vi "Dashboard Main.vi"() -> ()   [LabVIEW 2016]
uses:
  Vision/Camera Types.ctl
  Common Code/Drivetrain Encoder Settings.ctl
  Common Code/Drivetrain Encoder Values.ctl
  Common Code/Encoder Values.ctl
  Common Code/Drivetrain Status Cluster.ctl
  Common Code/Drivetrain Mode.ctl
  Common Code/Intake Auto States.ctl
  Common Code/Shooter Commands.ctl
  Common Code/Shot Type.ctl
  <vilib>/Rock Robotics/WPI/Camera/WPI_CameraSettings Read MJPG.ctl
  <vilib>/Rock Robotics/WPI/Camera/WPI_CameraImageSize.ctl
  Common Code/Goal Vision Packet.ctl
  Common Code/Auton Command Cluster.ctl
  Common Code/Auton File Lists.ctl
  <vilib>/Analysis/Matrix/Datatypes/RealMatrix.ctl
  Common Code/Climber Settings.ctl
  Common Code/PDP Device Currents.ctl
  Common Code/Drivetrain Settings.ctl
  Common Code/PID Gains.ctl
  Common Code/Input Modifier.ctl
  Common Code/Robot Status Cluster.ctl
  <vilib>/Rock Robotics/WPI/DriverStation/WPI_DriverStationRobotMode2.ctl
  <vilib>/Rock Robotics/WPI/DriverStation/WPI_DriverStationAllianceInfo.ctl
  <vilib>/Rock Robotics/WPI/DriverStation/WPI_DriverStationPositionInfo.ctl
  Common Code/LED Dashboard.ctl
  Common Code/Shooter Presets.ctl
  Common Code/Auto Agitator Settings.ctl
  Common Code/Shooter Motor Operational Status .ctl
  Common Code/Intake Presets.ctl
  Common Code/Shooter Status Cluster.ctl
  Common Code/Shooter Modes.ctl
  Common Code/Intake Status Cluster.ctl
  Common Code/Intake Modes.ctl
  Common Code/Intake Trip States.ctl
  Common Code/Load State.ctl
  Common Code/Unload Mode.ctl
  Common Code/Gear Vision Packet.ctl
  <vilib>/vision/Image Controls.llb/IMAQ Image.ctl
  Common Code/Dashboard Control Data.ctl
  Common Code/Vision Target Packet.ctl
  Common Code/LED Global Data.ctl
  Common Code/Robot Name.ctl
  Common Code/Dashboard Display Data.ctl
  Common Code/Climb Status Cluster.ctl
  Common Code/PDP Status Cluster.ctl
  Common Code/LED Status Cluster.ctl
  Common Code/PIXY Vision Packet.ctl
  Common Code/Utilities/Change Detect Int.vi
  <vilib>/Rock Robotics/WPI/Dashboard/WPI_DashboardLogging Global.vi
  <vilib>/Utility/inputDevices.llb/keyboardAcquire.vi
  <vilib>/vision/NI_Vision_Development_Module.lvlib
  <vilib>/Analysis/Matrix/NI_Matrix.lvlib
  <vilib>/picture/3D Picture Control/NI_3D Picture Control.lvlib
panel:
  out "Gear Vision Packet":T1
  out "Gear Front Cam":T2
  in  "Gear LED Color":T3={"Hue"={107.81818389892578, 139.81818389892578}, "Sat"={176.07142857142858, 255.0}, "Val"={40.53571428571429, 255.0}} {"Hue" scale=0.0..255.0 scale format="%#_3g"}
  in  "Gear Camera Type":T4=enum."1013"
  in  "Line Border 2":cluster{"Top":dbl, "Bottom":dbl}={"Top"=6.0, "Bottom"=1.0}
  out "DS TCP":T5
  in  "stop":bool
  in  "Rec Mode":enum32{"Stop", "Record", "Playback"}(radio)
  in  "TCP":refnum<k5>
  out "Robot IP":string
  out "Image Message":string="Timeout in Camera Communications"
  in  "Dashboard Tab":T6(tab)
  out "Pusher Activated?":bool
  out "Match Time\n(seconds)":dbl
  out "Climber Power":dbl(slide) scale=-1.0..1.0
  out "Match Time":string
  out "Current Auto Queue":string
  out "Gear?":bool
  out "back":u32(colorbox)
  out "front":u32(colorbox)
  out "Climber Tripped":bool
  out "Creep Mode?":bool
  out "Trigger Power":dbl(slide) scale=-1.0..1.0
  out "Intake Power":dbl(slide) scale=-1.0..1.0
  out "Current RPM":dbl
  out "Target RPM":dbl
  out "RPM Reached?":bool
  out "Vision Aligned?":bool
  out "Center":dbl(slide) scale=-200.0..200.0
  out "Right":dbl(slide) scale=-200.0..200.0
  out "Left":dbl(slide) scale=-200.0..200.0
  out "Target Angle Difference":dbl
  out "Distance from Target":dbl
  out "Target Found?":bool
  in  "Camera Mode 2":u16(ring) items=["Camera Off", "USB Camera SW", "USB Camera HW", "IP Camera"]
  in  "Camera Mode":u16(ring) items=["Camera Off", "USB Camera SW", "USB Camera HW", "IP Camera"]
  out "Front Camera Display":T2(plugin-control)
  out "Camera Info":cluster{"Mbps LED":bool, "Mbps":dbl, "fps":dbl} {"fps" format="%#.1g"; "Mbps" format="%#.1g"}
  out "RPM":cluster{dbl, dbl}(knob)={0.0, 114.36688146524764} scale=0.0..5000.0
  out "Traction":bool
  out "Brakes":bool
  out "Center Wheel":bool caption="Brakes"
  out "Pressure":dbl(slide) scale=0.0..120.0
  out "Wings":bool
  out "Gyro":cluster{dbl, dbl}(knob)={0.0, 101.11394868147904} scale=0.0..360.0
  out "Intake":bool
  out "Shooter":bool
  out "Shooter State":T7
  out "Shot Type":T8=enum."Dist Shot"
  out "Gear":bool
  out "Hood Down?":bool
  out "Complete Gear Load":bool
  out "Forward Tripped?":bool
  out "Backward Tripped?":bool
  out "Intake State":T9
  out "Camera Info 3":cluster{"Mbps LED":bool, "Mbps":dbl, "fps":dbl} {"fps" format="%#.1g"; "Mbps" format="%#.1g"}
  out "Robot":picture
  out "Doors Open?":bool
  out "Gear Cam":T2(plugin-control)
  in  "Drivetrain Settings":T10={"Gyro Tolerance"=1.5, "Gyro Steer PID Gains"={"proportional gain (Kc)"=0.03, "integral time (Ti, min)"=0.01, "derivative time (Td, min)"=0.0}, "Y Power Multiplier"=6.0, "Turn Power Multiplier"=5.0, "Gyro Output"=0.85, "Creep Rate"=0.4, "Distance Drive PID Gains"={"proportional gain (Kc)"=1.0, "integral time (Ti, min)"=0.01, "derivative time (Td, min)"=0.0}, "Distance Tolerance"=1.4999999999999998, "Distance Output"=0.85, "Strafe Threshold"=0.4, "Strafe Correct"=FALSE, "Strafe Tolerance"=0.0, "Translate Drive PID Gains"={"proportional gain (Kc)"=1.0, "integral time (Ti, min)"=0.01, "derivative time (Td, min)"=0.0}, "Strafe Output"=0.0, "SC Right"=0.85, "SC Left"=0.85, "Use Gyro"=FALSE, "Constant Power"=FALSE, "Strafe Power"=0.0, "Input Modifier"=enum."None", "SCR Delay"=0.85, "SCL Delay"=0.85} {"Translate Drive PID Gains"."derivative time (Td, min)" format="%.3f"; "Translate Drive PID Gains"."integral time (Ti, min)" format="%.3f"; "Translate Drive PID Gains"."proportional gain (Kc)" format="%.3f"; "Distance Drive PID Gains"."derivative time (Td, min)" format="%.3f"; "Distance Drive PID Gains"."integral time (Ti, min)" format="%.3f"; "Distance Drive PID Gains"."proportional gain (Kc)" format="%.3f"; "Turn Power Multiplier" scale=0.0..6.0; "Y Power Multiplier" scale=0.0..6.0; "Gyro Steer PID Gains"."derivative time (Td, min)" format="%.3f"; "Gyro Steer PID Gains"."integral time (Ti, min)" format="%.3f"; "Gyro Steer PID Gains"."proportional gain (Kc)" format="%.3f"}
  in  "Zero Gyro":bool
  in  "Drivetrain Encoder Settings":T13
  out "Drivetrain Encoder Values":T14
  out "Drivetrain Status Cluster":T16={"Y (Throttle)"=0.0, "X (Steer)"=0.0, "Z (Strafe)"=0.0, "Heading Target"=0.0, "Center Piston Down?"=FALSE, "Traction?"=FALSE, "Gyro Steer Finished?"=FALSE, "Distance Drive Finished?"=FALSE, "Gyro"=0.0, "Distance Target"=0.0, "Y Max Output"=0.0, "Y Min Output"=0.0, "X Max Output"=0.0, "X Min Output"=0.0, "Z Max Output"=0.0, "Z Min Output"=0.0, "Translation Target"=0.0, "Translation Drive Finished?"=FALSE, "PID Auto Drive Finished?"=FALSE, "Brake?"=FALSE, "Vision Aligned?"=FALSE, "Creep Mode Engaged?"=FALSE, "Drivetrain Mode"=enum."Gyro Steer", "Gear Vision Aligned?"=FALSE} {"Gyro" scale=180.0..-180.0}
  out "Intake Status Cluster":T18={"Roller Power"=0.0, "Intake Mode"=enum."Manual", "Intake Auto State"=enum."Idle", "Backward Tripped?"=FALSE, "Forward Tripped?"=FALSE, "Intake Current Trip State"=enum."Normal", "Gear Flap Open"=FALSE, "Doors Open"=FALSE, "Traction for Gear?"=FALSE, "Current"=0.0, "Intake Down?"=FALSE, "Gear Loaded"=FALSE, "Pusher Activated"=FALSE, "Gear Load State"=enum."Idle", "Unload Mode"=enum."None", "Unloading Gear?"=FALSE}
  out "Shooter Status Cluster":T23={"Current RPM"=0.0, "Trigger Power"=0.0, "Shooter Mode"=enum."Auto", "Shot Type"=enum."Dist Shot", "Shooter State"=enum."Idle ", "Target RPM"=0.0, "Hood Down?"=FALSE, "RPM Reached?"=FALSE, "User Inputed RPM"=0.0} {"Current RPM" scale=0.0..5000.0}
  in  "Intake Presets":T25
  out "Motor Operational Status":T26
  in  "Auto Agitator":T27
  in  "Shooter Presets":T28
  out "Distance Shots":T29
  in  "Particles":dbl=5.0
  in  "Camera Settings":T30={"fps"=30, "compression"=30, "Image Size"=enum."320x240", "Config Shown"=FALSE}
  out "Original Image":T2(plugin-control)
  in  "Camera Type":T4=enum."1013"
  in  "Line Border":cluster{"Top":dbl, "Bottom":dbl}={"Top"=6.0, "Bottom"=1.0}
  in  "Use Calibration":bool=TRUE
  in  "Score Cutoff %":dbl=70.0
  out "Qualified Particles":i32
  in  "LED Color":T3={"Hue"={107.81818389892578, 139.81818389892578}, "Sat"={176.07142857142858, 255.0}, "Val"={40.53571428571429, 255.0}} {"Hue" scale=0.0..255.0 scale format="%#_3g"}
  out "Results":T32 {"Score" format="%#_3g"; "Pixels"."Rectangle"."Numeric 5" format="%#_3g"; "Pixels"."Rectangle"."Numeric 3" format="%#_3g"; "Pixels"."Rectangle"."Numeric 2" format="%#_3g"; "Pixels"."Rectangle"."Numeric" format="%#_3g"; "Normalized"."Rectangle"."Numeric 5" format="%#_2g"; "Normalized"."Rectangle"."Numeric 3" format="%#_2g"; "Normalized"."Rectangle"."Numeric 2" format="%#_2g"; "Normalized"."Rectangle"."Numeric" format="%#_2g"; "Normalized"."Center"."?" format="%#_3g"; "Normalized"."Center"."?" format="%#_3g"; "Distance (ft)" format="%#_3g"}
  out "Masked Image":T2(plugin-control)
  out "Goal Vision Packet":T33
  in  "Vision Timeout":dbl=70.0
  out "Gear Results":T32 {"Score" format="%#_3g"; "Pixels"."Rectangle"."Numeric 5" format="%#_3g"; "Pixels"."Rectangle"."Numeric 3" format="%#_3g"; "Pixels"."Rectangle"."Numeric 2" format="%#_3g"; "Pixels"."Rectangle"."Numeric" format="%#_3g"; "Normalized"."Rectangle"."Numeric 5" format="%#_2g"; "Normalized"."Rectangle"."Numeric 3" format="%#_2g"; "Normalized"."Rectangle"."Numeric 2" format="%#_2g"; "Normalized"."Rectangle"."Numeric" format="%#_2g"; "Normalized"."Center"."?" format="%#_3g"; "Normalized"."Center"."?" format="%#_3g"; "Distance (ft)" format="%#_3g"}
  out "Gear Qualified Particles":i32
  in  "Gear Score Cutoff %":dbl=70.0
  in  "Gear Use Calibration":bool=TRUE
  out "Gear Original Image":T2(plugin-control)
  out "Gear Masked Image":T2(plugin-control)
  in  "Particles 2":dbl=5.0
  in  "Gear Camera Settings":T30={"fps"=30, "compression"=30, "Image Size"=enum."320x240", "Config Shown"=FALSE}
  in  "Gear Vision Packet 2":T1
  out "Auton File Lists":T34
  out "Auton Command Cluster":T35
  in  "Auton Presets":cluster{"Start Position":dbl}
  in  "LEDs":T36
  out "Robot Status Cluster":T37
  in  "Robot Photos Folder":path=path "C:/Users/Team624/Desktop/SteamyRobot/Dashboard/Dashboard Nautilus"
  out "Climber Current Tripped":bool
  in  "Climber Settings":T41
  in  "Pressure M":dbl
  in  "Pressure B":dbl
  out "Pressure":dbl
  out "Pressure Voltage":dbl
  out "Total Current":dbl
  out "PDP Currents":T42
  out "Status Info":T43
  out "Control Info":T44
  out "Robot Metrics":T45
  out "Shooter RPM History":dbl(graph)
  in  "Open in Excel":bool
  in  "Save":bool
  in  "Load":bool
  out "DumbDashMessage":string
  # "CRyptonite Robotics DumbDashboard 2k17"
  # "Drivetrain"
  # "Collection"
  # "Drivetrain Speeds"
  # "Driver\nA0 - none\nA1 - Throttle\nA2 - Strafe Left\nA3 - Strafe Right\nA4 - Turn\nA5 - none\n\nB0 - Vision Align (Hold)\nB1 - none\nB2 - none\nB3 - Brakes (Hold)\nB4 - Creep Mode (Hold)\nB5 - Traction (Toggle)\nB6 - none\nB7 - none\nB8 - none\nB9 - none\n\nU - none\nD - none\nL - Gyro Steer Left (Hold)\nR - Gyro Steer Right (Hold)"
  # "Manipulator\nA0 - none\nA1 - Manual Shooter Power\nA2 - Outtake\nA3 - Intake\nA4 - none\nA5 - Manual Trigger Power\n\nB0 - Shoot (Hold)\nB1 - Change Intake Mode (Toggle)\nB2 - Warmup Shooter (Hold)\nB3 - Change Shooter Mode (Toggle)\nB4 - Engage Traction for Gear (Hold)\nB5 - Manual Hood (Toggle)\nB6 - Agitator (Hold)\nB7 - Climb\nB8 - Open Gear Flap (Hold)\nB9 - Open Wings (Hold)\n\nU - none\nD - none\nL - Distance Shot Type (1 Way Toggle)\nR - Key Shot Type (1 Way Toggle"
  # "A2"
  # "A3"
  # "B4"
  # "B5"
  # "B6"
  # "B7"
  # "B3"
  # "U"
  # "B2"
  # "B1"
  # "L"
  # "R"
  # "A5"
  # "A1"
  # "B0"
  # "D"
  # "A0"
  # "A4"
  # "B8"
  # "B9"
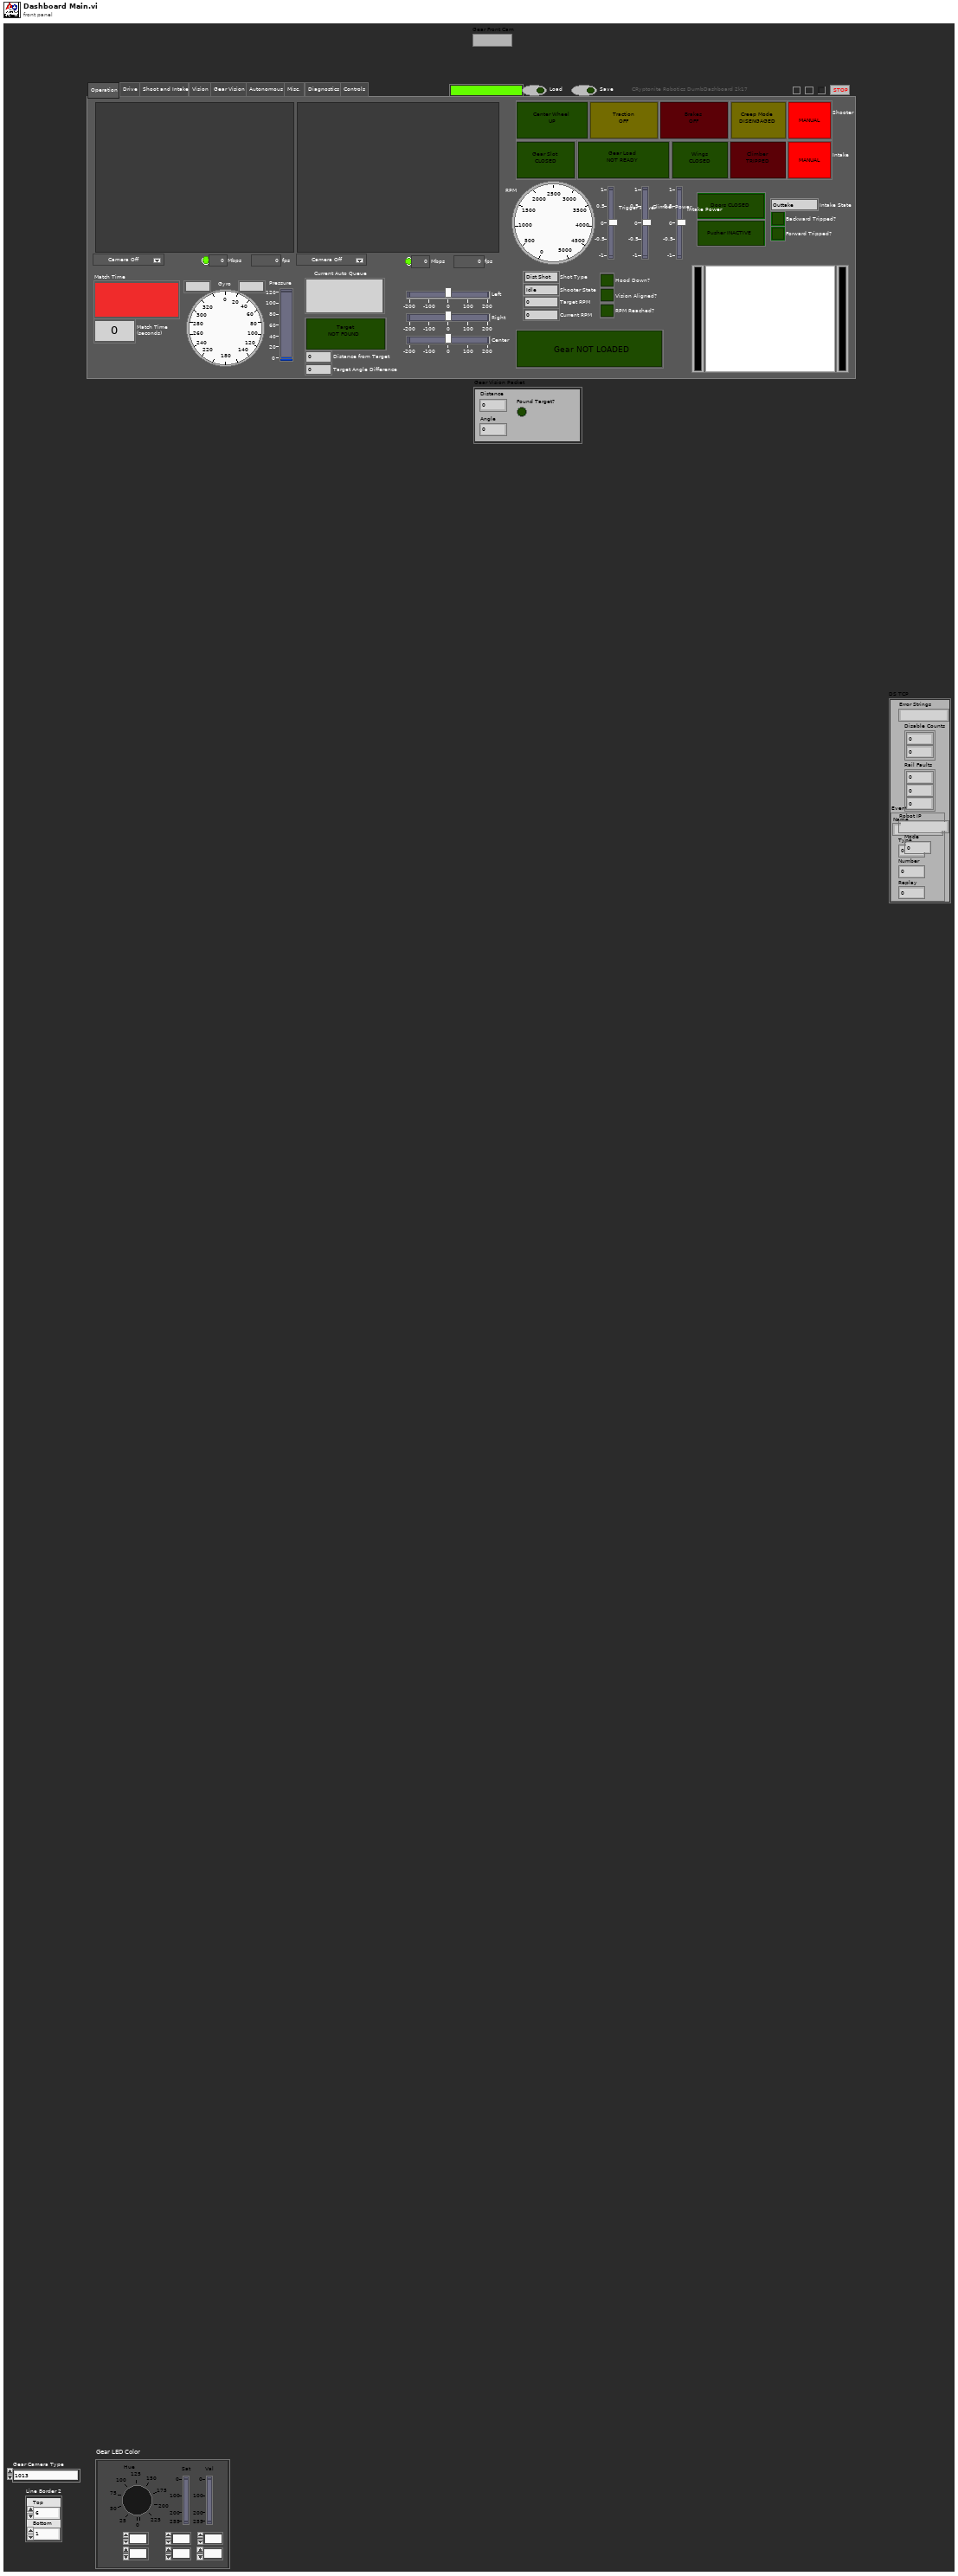
[diagram p1: front panel]
types:
  T1 = typedef "Gear Vision Packet.ctl" = cluster{"Distance":dbl, "Angle":dbl, "Found Target?":bool}
  T2 = typedef "IMAQ Image.ctl" = refnum<image>
  T3 = cluster{"Hue":cluster{dbl, dbl}, "Sat":cluster{dbl, dbl}, "Val":cluster{dbl, dbl}}
  T4 = typedef "Camera Types.ctl" = enum16{"206", "1011", "1013", "MS HD3000 square", "MS HD3000 640x480"}
  T5 = cluster{"Error Strings":string, "Disable Counts":cluster{u16, u16}, "Rail Faults":cluster{u16, u16, u16}, "Robot IP":string, "Mode":u8, "Event Info":cluster{"Name":string, "Type":u8, "Number":u16, "Replay":u8}}
  T6 = enum32{"Operation", "Drive", "Shoot and Intake", "Vision", "Gear Vision", "Autonomous", "Misc.", "Diagnostics", "Controls"}
  T7 = typedef "Shooter Commands.ctl" = enum16{"Idle ", "Warmup ", "Shoot"}
  T8 = typedef "Shot Type.ctl" = enum16{"Vision Shot", "Dist Shot", "Key Shot"}
  T9 = typedef "Intake Auto States.ctl" = enum16{"Outtake", "Idle", "Intake", "Intake Pull Up"}
  T10 = typedef "Drivetrain Settings.ctl" = cluster{"Gyro Tolerance":dbl, "Gyro Steer PID Gains":T11, "Y Power Multiplier":dbl, "Turn Power Multiplier":dbl, "Gyro Output":dbl, "Creep Rate":dbl, "Distance Drive PID Gains":T11, "Distance Tolerance":dbl, "Distance Output":dbl, "Strafe Threshold":dbl, "Strafe Correct":bool, "Strafe Tolerance":dbl, "Translate Drive PID Gains":T11, "Strafe Output":dbl, "SC Right":dbl, "SC Left":dbl, "Use Gyro":bool, "Constant Power":bool, "Strafe Power":dbl, "Input Modifier":T12, "SCR Delay":dbl, "SCL Delay":dbl}
  T11 = typedef "PID Gains.ctl" = cluster{"proportional gain (Kc)":dbl, "integral time (Ti, min)":dbl, "derivative time (Td, min)":dbl}
  T12 = typedef "Input Modifier.ctl" = enum16{"None", "Square", "Cube"}
  T13 = typedef "Drivetrain Encoder Settings.ctl" = cluster{"Left Tick Constant":dbl, "Right Tick Contant":dbl, "Reset Encoders":bool, "Center Tick Constant":dbl}
  T14 = typedef "Drivetrain Encoder Values.ctl" = cluster{"Left Encoder":T15, "Center Encoder":T15, "Right Encoder":T15}
  T15 = typedef "Encoder Values.ctl" = cluster{"Distance":dbl, "Speed":dbl, "Tick":dbl}
  T16 = typedef "Drivetrain Status Cluster.ctl" = cluster{"Y (Throttle)":dbl, "X (Steer)":dbl, "Z (Strafe)":dbl, "Heading Target":dbl, "Center Piston Down?":bool, "Traction?":bool, "Gyro Steer Finished?":bool, "Distance Drive Finished?":bool, "Gyro":dbl, "Distance Target":dbl, "Y Max Output":dbl, "Y Min Output":dbl, "X Max Output":dbl, "X Min Output":dbl, "Z Max Output":dbl, "Z Min Output":dbl, "Translation Target":dbl, "Translation Drive Finished?":bool, "PID Auto Drive Finished?":bool, "Brake?":bool, "Vision Aligned?":bool, "Creep Mode Engaged?":bool, "Drivetrain Mode":T17, "Gear Vision Aligned?":bool}
  T17 = typedef "Drivetrain Mode.ctl" = enum16{"Gear Vision Align", "Manual", "Gyro Steer", "Distance Drive", "Translate Drive", "Goal Vision Align", "PID Drive"}
  T18 = typedef "Intake Status Cluster.ctl" = cluster{"Roller Power":dbl, "Intake Mode":T19, "Intake Auto State":T9, "Backward Tripped?":bool, "Forward Tripped?":bool, "Intake Current Trip State":T20, "Gear Flap Open":bool, "Doors Open":bool, "Traction for Gear?":bool, "Current":dbl, "Intake Down?":bool, "Gear Loaded":bool, "Pusher Activated":bool, "Gear Load State":T21, "Unload Mode":T22, "Unloading Gear?":bool}
  T19 = typedef "Intake Modes.ctl" = enum16{"Manual", "Auto"}
  T20 = typedef "Intake Trip States.ctl" = enum16{"Normal", "Backward Tripped", "Forward Tripped"}
  T21 = typedef "Load State.ctl" = enum16{"Idle", "Open Flap", "Ready Close", "Ready Far"}
  T22 = typedef "Unload Mode.ctl" = enum16{"None", "Close", "Far"}
  T23 = typedef "Shooter Status Cluster.ctl" = cluster{"Current RPM":dbl, "Trigger Power":dbl, "Shooter Mode":T24, "Shot Type":T8, "Shooter State":T7, "Target RPM":dbl, "Hood Down?":bool, "RPM Reached?":bool, "User Inputed RPM":dbl}
  T24 = typedef "Shooter Modes.ctl" = enum16{"Auto", "Manual"}
  T25 = typedef "Intake Presets.ctl" = cluster{"Intake Speed ":dbl, "Outake Speed":dbl, "Current Trip Delay":dbl, "Max Current":dbl, "Gear Outtake Motor Delay":dbl, "Gear Intake Motor Delay":dbl, "Gear Intake Pull Up Speed":dbl, "Pusher Delay":dbl, "Release Delay":dbl, "Close Release Delay":dbl}
  T26 = typedef "Shooter Motor Operational Status .ctl" = cluster{"Sensor Velocity ":dbl, "Encoder Position":dbl, "Encoder Velocity ":dbl, "Encoder Index Count":dbl, "Analog In":dbl, "Analog In Velocity":dbl, "Battery Voltage":dbl, "Current":dbl, "Sensor Position":dbl, "Vel Div 4":bool, "Encoder A Pin State":bool, "Encoder B Pin State":bool, "Encoder Index Pin State":bool, "Pulse Width Velocity ":dbl}
  T27 = typedef "Auto Agitator Settings.ctl" = cluster{"Enable Auto Agitation":bool, "Continuous Stir":bool, "Continuous Intake":bool, "Alternate In/Outtake":bool, "Wing Delay":dbl, "Stir Delay":dbl, "Intake Delay":dbl, "Wing On Time":dbl, "Wing Off Time":dbl, "Stir On Time":dbl, "Stir Off Time":dbl, "Intake On Time":dbl, "Intake Off Time":dbl, "Stir Power":dbl, "Intake Power":dbl, "Outtake Power":dbl, "Intake Run Time":dbl, "Outtake Run Time":dbl, "Wing$":bool, "Intake":bool, "Stirrer":bool}
  T28 = typedef "Shooter Presets.ctl" = cluster{"Key Shot":cluster{"RPM ":dbl, "Hood?":bool}, "Distance Shot":cluster{"RPM":dbl, "Hood?":bool}, "RPM Tolerance":dbl, "Unstuck Delay Time ":dbl, "Initial RPM Increase":dbl, "Warmup Delay":dbl, "Faster Time":dbl, "Shooter PID Gains":cluster{"P":dbl, "I":dbl, "D":dbl, "FF":dbl, "Ramp Rate":dbl, "I Zone":dbl}, "Unstuck Trigger Power":dbl, "Trigger Power":dbl, "Unstuck RPM":dbl, "Agitator Active Power":dbl, "Agitator Idle Power":dbl, "RPM Tuning Range":dbl, "RPM M Tuning Range":dbl}
  T29 = typedef "NI_Matrix.lvlib/RealMatrix.ctl" = dbl[][]
  T30 = typedef "WPI_CameraSettings Read MJPG.ctl" = cluster{"fps":i32, "compression":i32, "Image Size":T31, "Config Shown":bool}
  T31 = typedef "WPI_CameraImageSize.ctl" = enum16{"640x480", "320x240", "160x120", "Custom"}
  T32 = cluster{"Distance (ft)":dbl, "Score":dbl, "Normalized":cluster{"Center":cluster{dbl, dbl}, "Rectangle":cluster{"Numeric":dbl, "Numeric 2":dbl, "Numeric 3":dbl, "Numeric 5":dbl}}, "Pixels":cluster{"Center":cluster{dbl, dbl}, "Rectangle":cluster{"Numeric":dbl, "Numeric 2":dbl, "Numeric 3":dbl, "Numeric 5":dbl}}}
  T33 = typedef "Goal Vision Packet.ctl" = cluster{"Distance":dbl, "Angle":dbl, "Found Target?":bool}
  T34 = typedef "Auton File Lists.ctl" = cluster{"Current Queue":string, "General Scripts":string, "Movements":string}
  T35 = typedef "Auton Command Cluster.ctl" = cluster{"commandID":dbl, "maxTime":dbl, "distanceTarget":dbl, "headingTarget":dbl, "translationTarget":dbl, "ySpeed":dbl, "xSpeed":dbl, "zSpeed":dbl, "async":dbl, "shotType":dbl, "shootCommand":dbl, "rollerPower":dbl, "fillHopper?":dbl, "zeroGyro":dbl, "openGear":dbl, "traction?":dbl}
  T36 = typedef "LED Dashboard.ctl" = cluster{"Back":cluster{"Default":string, "Gear Ready Close":string, "Break On":string, "Gear Loaded":string, "Traction":string, "Climb":string, "Gear Ready Far":string, "Unload Gear":string, "Prime Unload":string}, "LEDOnTime":dbl, "LEDOffTime":dbl, "Front":cluster{"Default":string, "Traction":string, "Gear Ready Close":string, "Break On":string, "Gear Loaded":string, "Climb":string, "Gear Ready Far":string, "Unload Gear":string, "Prime Unload":string}}
  T37 = typedef "Robot Status Cluster.ctl" = cluster{"RobotMode":T38, "Alliance":T39, "Position":T40, "Match Time":dbl, "FMS?":bool}
  T38 = typedef "WPI_DriverStationRobotMode2.ctl" = enum16{"Autonomous Disabled", "Autonomous Enabled", "Teleop Disabled", "Teleop Enabled", "Disconnected", "Finish", "Test Disabled", "Test Enabled", "Emergency Stopped"}
  T39 = typedef "WPI_DriverStationAllianceInfo.ctl" = enum16{"Red", "Blue", "Invalid"}
  T40 = typedef "WPI_DriverStationPositionInfo.ctl" = enum16{"1", "2", "3"}
  T41 = typedef "Climber Settings.ctl" = cluster{"Climber Power":dbl, "Max Current":dbl, "Avoid Current Trip?":bool}
  T42 = typedef "PDP Device Currents.ctl" = cluster{"Drivetrain Left CIM 1":dbl, "Drivetrain Left CIM 2":dbl, "Drivetrain Left Mini CIM":dbl, "Drivetrain Right CIM 1":dbl, "Drivetrain Right CIM 2":dbl, "Drivetrain Right Mini CIM":dbl, "Drivetrain Center CIM 1":dbl, "Drivetrain Center CIM 2":dbl, "Shooter Motor 1":dbl, "Shooter Motor 2":dbl, "Climber Motor 1":dbl, "Climber Motor 2":dbl, "Intake Motor":dbl, "Trigger Motor":dbl, "Fans/Compressor":dbl}
  T43 = cluster{"Status bits":cluster{"Test Mode":bool, "Autonomous":bool, "Enabled":bool, "Code Start":bool, "Brownout":bool, "Reserved 2":bool, "Reserved 3":bool, "E-Stop":bool}, "Code Trace":cluster{"Disabled":bool, "TeleOp":bool, "Auto":bool, "Test":bool}, "Controller Type":enum16{"unknown", "cRIO", "roboRio"}, "Code?":enum16{"unknown", "noCode", "code"}, "Battery V":dbl}
  T44 = cluster{"Control Bits":cluster{"TestMode":bool, "Autonomous":bool, "Enabled":bool, "FMS Present":bool, bool, bool, bool, "E-Stop":bool}, "Team Station ":u8, "Countdown":sgl, "Joystick Values":cluster{"Axes":dbl[], "Buttons":bool[], "POVs":i16[]}[]}
  T45 = cluster{"Storage":cluster{"Disk Free":u64, "RAM Block":u32, "RAM free":u32}, "CPU Utilization":cluster{"CPU % ISR":sgl, "CPU % Time Crit":sgl, "CPU % Timed Str":sgl, "CPU % High":sgl, "CPU % Above":sgl, "CPU % Normal":sgl, "CPU % Low":sgl}, "CAN":cluster{"% Bus Utilization":sgl, "Bus Off Cnt":u32, "TX_FIFO Full Cnt":u32, "Receive Error Cnt":u8, "Transmit Error Cnt":u8}, "HID":cluster{"HID Outputs":u32, "Rumble Low":u16, "Rumble High":u16}[]}
  T46 = typedef "Image Type" = u32
  T47 = typedef "Particle Parameters" = i32
  T48 = cluster{"IDs":cluster{"RPC field ID":u16, "Unique ID":u16}, "String":string}
  T49 = enum32{"Drive", "Basic", "Custom", "Test", "Checklist", "Variables"}
  T50 = typedef "LED Global Data.ctl" = cluster{"Back":cluster{"Default":string, "Traction":string, "Gear Ready Close":string, "Break On":string, "Gear Loaded":string, "Climb":string, "Gear Ready Far":string, "Unload Gear":string, "Prime Unload":string}, "Front":cluster{"Default":string, "Traction":string, "Gear Ready Close":string, "Break On":string, "Gear Loaded":string, "Climb":string, "Gear Ready Far":string, "Unload Gear":string, "Prime Unload":string}, "LEDOnTime":dbl, "LEDOffTime":dbl}
  T51 = typedef "Dashboard Control Data.ctl" = cluster{"Drivetrain Settings":T10, "Intake Presets ":T25, "Shooter Presets":T28, "Vision Target Packet":T52, "Auton Presets":cluster{"Start Position":dbl}, "Drivetrain Encoder Values":T14, "Drivetrain Encoder Settings":cluster{"Left Tick Constant":dbl, "Right Tick Contant":dbl, "Reset Encoders":bool, "Center Tick Constant":dbl}, "Zero Gyro":bool, "Vision Timeout":dbl, "Pressure M":dbl, "Pressure B":dbl, "Auto Agitator":T27, "Climber Settings":T41, "LEDs":T50}
  T52 = typedef "Vision Target Packet.ctl" = cluster{"Robot Center":dbl, "Center X":dbl, "Center Y":dbl, "Angle":dbl, "Distance":dbl, "Found Target?":bool}
  T53 = cluster{cluster{dbl, dbl}, cluster{dbl, dbl}, cluster{dbl, dbl}}
  T54 = cluster{"Left":dbl, "Top":dbl, "Right":dbl, "Bottom":dbl}
  T55 = cluster{"Numeric":dbl, "Numeric 2":dbl, "Numeric 3":dbl, "Numeric 5":dbl}
  T56 = enum16{"0", "1", "2", "3", "4", "5", "6", "7", "8", "9", "A", "B", "C", "D", "E", "F", "G", "H", "I", "J", "K", "L", "M", "N", "O", "P", "Q", "R", "S", "T", "U", "V", "W", "X", "Y", "Z", "F1", "F2", "F3", "F4", "F5", "F6", "F7", "F8", "F9", "F10", "F11", "F12", "F13", "F14", "F15", "ADD", "BACK", "BACKSLASH", "CAPITAL", "COMMA", "DECIMAL", "DELETE", "DIVIDE", "DOWN", "END", "EQUALS", "ESCAPE", "GRAVE (`)", "HOME", "INSERT", "LBRACKET", "LCONTROL", "LEFT", "L ALT", "LSHIFT", "LWIN", "MINUS", "MULTIPLY", "NEXT", "NUMLOCK", "NUMPAD_0", "NUMPAD_1", "NUMPAD_2", "NUMPAD_3", "NUMPAD_4", "NUMPAD_5", "NUMPAD_6", "NUMPAD_7", "NUMPAD_8", "NUMPAD_9", "PAUSE", "PERIOD", "PRIOR (PG UP)", "RBRACKET", "RCONTROL", "RETURN", "RIGHT", "R ALT", "RSHIFT", "RWIN", "SCROLL", "SEMICOLON", "SLASH", "SPACE", "SUBTRACT", "TAB", "UP", "ENTER (num pad)", "' (quote)"}
  T57 = enum16{"0", "1", "2", "3", "4", "5", "6", "7", "8", "9", "A", "B", "C", "D", "E", "F", "G", "H", "I", "J", "K", "L", "M", "N", "O", "P", "Q", "R", "S", "T", "U", "V", "W", "X", "Y", "Z", "F1", "F2", "F3", "F4", "F5", "F6", "F7", "F8", "F9", "F10", "F11", "F12", "F13", "F14", "F15", "ADD", "BACK", "BACKSLASH", "CAPITAL", "COMMA", "DECIMAL", "DELETE", "DIVIDE", "DOWN", "END", "EQUALS", "ESCAPE", "GRAVE (`)", "HOME", "INSERT", "LBRACKET", "LCONTROL", "LEFT", "L ALT", "LSHIFT", "LWIN", "MINUS", "MULTIPLY", "NEXT", "NUMLOCK", "NUMPAD_0", "NUMPAD_1", "NUMPAD_2", "NUMPAD_3", "NUMPAD_4", "NUMPAD_5", "NUMPAD_6", "NUMPAD_7", "NUMPAD_8", "NUMPAD_9", "PAUSE", "PERIOD", "PRIOR (PG UP)", "RBRACKET", "RCONTROL", "RETURN", "RIGHT", "R ALT", "RSHIFT", "RWIN", "SCROLL", "SEMICOLON", "SLASH", "SPACE", "SUBTRACT", "TAB", "UP", "ENTER (num pad)", "' (quote)"}[]
  T58 = typedef "Dashboard Display Data.ctl" = cluster{"Climb Status Cluster":T59, "Drivetrain Status Cluster":T16, "Intake Status Cluster":T18, "Shooter Status Cluster":T23, "Drivetrain Encoder Values":T14, "Auton Command Cluster":T35, "Auton File Lists":T34, "Pressure":dbl, "Pressure Voltage":dbl, "Motor Operational Status":T26, "Vision Presets":T29, "Climber Current Tripped?":bool, "Gear?":bool, "PDP Status Cluster":T60, "Robot Status Cluster":T37, "LED Status Cluster":T61, "PIXY Vision Packet":T62}
  T59 = typedef "Climb Status Cluster.ctl" = cluster{"Climb Speed":dbl}
  T60 = typedef "PDP Status Cluster.ctl" = cluster{"Drivetrain Left CIM 1":dbl, "Drivetrain Left CIM 2":dbl, "Drivetrain Left Mini CIM":dbl, "Drivetrain Right CIM 1":dbl, "Drivetrain Right CIM 2":dbl, "Drivetrain Right Mini CIM":dbl, "Drivetrain Center CIM 1":dbl, "Drivetrain Center CIM 2":dbl, "Shooter Motor 1":dbl, "Shooter Motor 2":dbl, "Climber Motor 1":dbl, "Climber Motor 2":dbl, "Intake Motor":dbl, "Trigger Motor":dbl, "Fans/Compressor":dbl}
  T61 = typedef "LED Status Cluster.ctl" = cluster{"Front Red":bool, "Front Green":bool, "Front Blue":bool, "Back Red":bool, "Back Green":bool, "Back Blue":bool}
  T62 = typedef "PIXY Vision Packet.ctl" = cluster{"Objects":cluster{"Signature":u16, "X Position":u16, "Y Position":u16, "Width":u16, "Height":u16}[]}
  T63 = enum8{"Tele-Op Disabled", "Tele-Op Enabled", "Auto Disabled", "Auto Enabled", "Test Disabled", "Test Enabled", "Disconnected", "No Code", "E-Stop"}
  T64 = typedef "LVDateTimeRec.ctl" = cluster{"fractional second":dbl, "second":i32, "minute":i32, "hour":i32, "day of month":i32, "month":i32, "year":i32, "day of week":i32, "day of year":i32, "DST":i32}
  T65 = typedef "imagedata.ctl" = cluster{"image type":i32, "image depth":i32, "image":u8[], "mask":u8[], "colors":u32[], "Rectangle":cluster{"left":i16, "top":i16, "right":i16, "bottom":i16}}
  T66 = cluster{"Image Size":bool, "Image Type":bool, "Pixel Value":bool, "ROI Information":bool, "Zoom Factor":bool}
  T67 = typedef "DumbDash Control.ctl" = cluster{"Name":string, "Ref":refnum<vi>, "Type":T68}
  T68 = typedef "DumbDash Control Type.ctl" = enum16{"Invalid", "Number", "Boolean", "String"}
  T69 = typedef "Robot Name.ctl" = u16
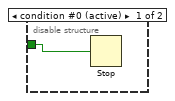
[diagram p5: hidden frame]
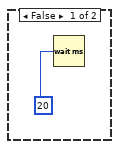
[diagram p6: hidden frame]
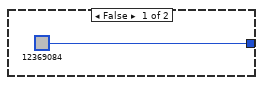
[diagram p9: hidden frame]
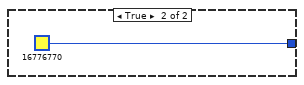
[diagram p10: hidden frame]
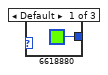
[diagram p13: hidden frame]
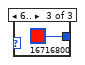
[diagram p14: hidden frame]
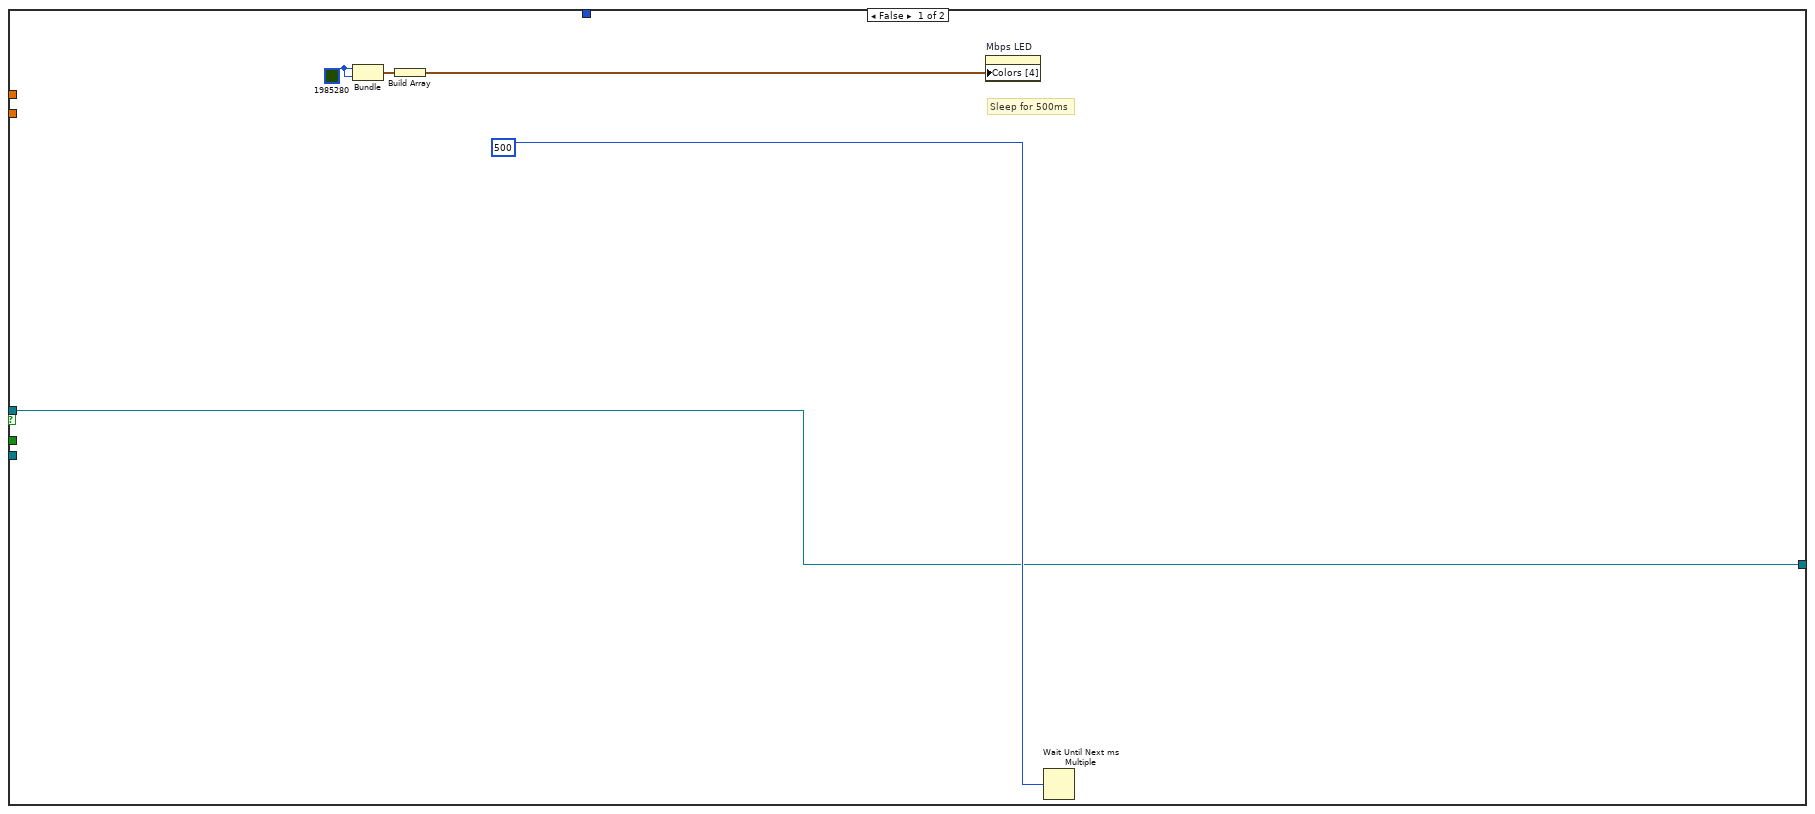
[diagram p15: hidden frame]
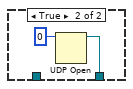
[diagram p16: hidden frame]
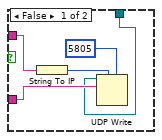
[diagram p17: hidden frame]
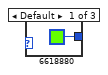
[diagram p19: hidden frame]
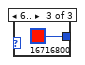
[diagram p20: hidden frame]
diagram:
  w3 = T46 4 items=["Grayscale (U8)", "Grayscale (I16)", "Grayscale (SGL)", "Complex (CSG)", "RGB (U32)", "HSL (U32)", "RGB (U64)"] ("Image Type")
  w6 = T46 4 items=["Grayscale (U8)", "Grayscale (I16)", "Grayscale (SGL)", "Complex (CSG)", "RGB (U32)", "HSL (U32)", "RGB (U64)"] ("Image Type")
  w9 = T46 0 items=["Grayscale (U8)", "Grayscale (I16)", "Grayscale (SGL)", "Complex (CSG)", "RGB (U32)", "HSL (U32)", "RGB (U64)"] ("Image Type")
  w14 = enum32{"Stop", "Record", "Playback"}."Stop" ("Rec Mode")
  w21 = T47[] [48, 35, 4, 5, 6, 7, 0, 1] items=["Center of Mass X", "Center of Mass Y", "First Pixel X", "First Pixel Y", "Bounding Rect Left", "Bounding Rect Top", "Bounding Rect Right", "Bounding Rect Bottom", "Max Feret Diameter Start X", "Max Feret Diameter Start Y", "Max Feret Diameter End X", "Max Feret Diameter End Y", "Max Horiz. Segment Length Left", "Max Horiz. Segment Length Right", "Max Horiz. Segment Length Row", "-", "Bounding Rect Width", "Bounding Rect Height", "Bounding Rect Diagonal", "Perimeter", "Convex Hull Perimeter", "Holes' Perimeter", "Max Feret Diameter", "Equivalent Ellipse Major Axis", "Equivalent Ellipse Minor Axis", "Equivalent Ellipse Minor Axis (Feret)", "Equivalent Rect Long Side", "Equivalent Rect Short Side", "Equivalent Rect Diagonal", "Equivalent Rect Short Side (Feret)", "Average Horiz. Segment Length", "Average Vert. Segment Length", "Hydraulic Radius", "Waddel Disk Diameter", "-", "Area", "Holes' Area", "Particle & Holes' Area", "Convex Hull Area", "Image Area", "-", "Number of Holes", "Number of Horiz. Segments", "Number of Vert. Segments", "-", "Orientation", "Max Feret Diameter Orientation", "-", "% Area/Image Area", "% Area/(Particle & Holes' Area)", "Ratio of Equivalent Ellipse Axes", "Ratio of Equivalent Rect Sides", "-", "Elongation Factor", "Compactness Factor", "Heywood Circularity Factor", "Type Factor", "-", "Sum X", "Sum Y", "Sum XX", "Sum XY", "Sum YY", "Sum XXX", "Sum XXY", "Sum XYY", "Sum YYY", "-", "Moment of Inertia XX", "Moment of Inertia XY", "Moment of Inertia YY", "Moment of Inertia XXX", "Moment of Inertia XXY", "Moment of Inertia XYY", "Moment of Inertia YYY", "Norm. Moment of Inertia XX", "Norm. Moment of Inertia XY", "Norm. Moment of Inertia YY", "Norm. Moment of Inertia XXX", "Norm. Moment of Inertia XXY", "Norm. Moment of Inertia XYY", "Norm. Moment of Inertia YYY", "Hu Moment 1", "Hu Moment 2", "Hu Moment 3", "Hu Moment 4", "Hu Moment 5", "Hu Moment 6", "Hu Moment 7"] ("Pixel Measurements")
  w25 = T48 {"IDs"={"RPC field ID"=0, "Unique ID"=0}, "String"=""}  # RPC Response
  w31 = 491  # min tab size
  w30 = 1.333  # min tab size
  (unwired) "This VI has seven parallel loops for different tasks and a bit of initialization code that runs just once.\n\nTypical dashboard extensions only need to edit the panel. Adding new indicators or controls simply involves placing them on the panel in the Operations tab and naming them the same as the SmartDashboard variable on the robot\n\nIf the display needs to process the data before display, loop one is an example of doing that for the joysticks and motors.\n\nIf you want customize the video display or perform processing on it, loop two is where that takes place.\n\nOther loops should not need to be modified. They are pretty standard, and document the task they perform."  # Documentation
  w46 = T46 4 items=["Grayscale (U8)", "Grayscale (I16)", "Grayscale (SGL)", "Complex (CSG)", "RGB (U32)", "HSL (U32)", "RGB (U64)"] ("Image Type")
  # "displays ur stuff on the dashboard"
  # "sends ur stuff to the dashboard"
  # "Vision code"
  # "Controls for Test Mode, Camera Settings, etc."
  # "Additional UI Initialization"
  # "Loop 6. Animation for background of window during playback and record"
  # "Fires each time robot IP\nchanges, simulator does this"
  # "Fires each time window\ndocking changes."
  # "Collects all controls and indicators\nin the Basic and Custom tab.\nIf you need to bind additional controls,\nadd their references. You can extend the\nenum constant or use an integer."
  # "The remaining code below this line typically doesn't need to be modified."
  # "Loop 4. Process UI events related to test mode, checklist, and camera settings"
  # "Terminals of controls and indicators that are bound to the smart dashboard by name.\nYou can place the terminals anywhere you like and even read data from them.\nYou bind controls by adding the control reference to the array on the left. The subVI will\ndo this for the contents of a tab, and you can do it for individual items too, as shown with\nthe LED. To create get the reference, right-click and Create>>Reference."
  # "Loop 3. Wait until the robot response provides\n the Robot IP address.\nOnce known, bind controls and\nvariables with the same names."
  # "Loop 5. Adjusts placement onscreen, hides the titlebar, etc."
  # "Loop 1. Receive various data streams from Driver Station, update joystick, motors, and more complex displays that don't easily bind to variables."
  n1 = control-ref of="Rec Mode"() -> ()  [unwired: 1 out]
  n2 = control-ref of="Dashboard Tab"() -> ()  [unwired: 1 out]
  n3 = control-ref of="Dashboard Tab"() -> (w34:refnum<vi>)
  n4 = property class="VI" props=["Front Panel.Closeable"]() -> (reference out=w15:refnum<vi>)  [unwired: 2 in, 2 out]
  n5 = Bundle("min tab size"=w31, "min tab size"=w30) -> ()  [unwired: 1 in, 1 out]
  n6 = Create User Event(user event datatype=w25) -> (user event=w20:refnum<user-event>)  [unwired: 1 in, 1 out]
  n7 = Obtain Notifier(name (unnamed)="Window Mode", notification data type=TRUE) -> (notifier out=w24:refnum<notifier>)  [unwired: 2 in, 2 out]
  n8 = call <vilib>:"Get Tab Control Refs.vi"("Page Index"=T49."Basic" ("Dashboard Tab"), "TabControl in"=w34) -> ("ControlsOnPage"=w19:refnum<vi>[])  [unwired: 9 in]
  n9 = call <vilib>:"Get Tab Control Refs.vi"("Page Index"=T49."Custom" ("Dashboard Tab"), "TabControl in"=w34) -> ("ControlsOnPage"=w33:refnum<vi>[])  [unwired: 9 in]
  n10 = Obtain Notifier(name (unnamed)="Robot IP Update", notification data type="IP Addr" ("name (unnamed)")) -> (notifier out=w27:refnum<notifier>)  [unwired: 2 in, 2 out]
  n11 = Build Array (concatenate)(w19, w33) -> (w32:refnum<vi>[])
  n12 = while {
    stop <- FALSE stop-if-true
    n13 = Unbundle By Name("LEDs") -> ("Front.Default"=w71:string, "Front.Traction"=w70:string, "Front.Gear Ready Close"=w69:string, "Front.Break On"=w68:string, "Front.Gear Loaded"=w67:string, "Front.Climb"=w66:string, "Front.Gear Ready Far"=w65:string, "Front.Unload Gear"=w64:string, "Back.Default"=w63:string, "Back.Gear Ready Close"=w62:string, "Back.Break On"=w61:string, "Back.Gear Loaded"=w60:string, "Back.Traction"=w59:string, "Back.Climb"=w58:string, "Back.Gear Ready Far"=w57:string, "Back.Unload Gear"=w56:string, "LEDOnTime"=w55:dbl, "LEDOffTime"=w54:dbl, "Back.Prime Unload"=w47:string, "Front.Prime Unload"=w48:string)
    n14 = flat-sequence {
      tunnel: "Zero Gyro" -> [w88]
      tunnel: [w88] -> w73
      frame #0 {
      }
      frame #1 {
        n15 = local write "Zero Gyro"(FALSE ("Zero Gyro")) -> ()
      }
    }
    n16 = Bundle By Name(cluster=T50 {"Back"={"Default"="", "Traction"="", "Gear Ready Close"="", "Break On"="", "Gear Loaded"="", "Climb"="", "Gear Ready Far"="", "Unload Gear"="", "Prime Unload"=""}, "Front"={"Default"="", "Traction"="", "Gear Ready Close"="", "Break On"="", "Gear Loaded"="", "Climb"="", "Gear Ready Far"="", "Unload Gear"="", "Prime Unload"=""}, "LEDOnTime"=0.0, "LEDOffTime"=0.0} ("LEDs"), "Front.Default"=w71, "Front.Traction"=w70, "Front.Gear Ready Close"=w69, "Front.Break On"=w68, "Front.Gear Loaded"=w67, "Front.Climb"=w66, "Front.Gear Ready Far"=w65, "Front.Unload Gear"=w64, "Back.Default"=w63, "Back.Gear Ready Close"=w62, "Back.Break On"=w61, "Back.Gear Loaded"=w60, "Back.Traction"=w59, "Back.Climb"=w58, "Back.Gear Ready Far"=w57, "Back.Unload Gear"=w56, "LEDOnTime"=w55, "LEDOffTime"=w54, "Back.Prime Unload"=w47, "Front.Prime Unload"=w48) -> (w53:T50)
    n17 = Bundle By Name(cluster=T51 {"Drivetrain Settings"={"Gyro Tolerance"=1.5, "Gyro Steer PID Gains"={"proportional gain (Kc)"=1.0, "integral time (Ti, min)"=0.01, "derivative time (Td, min)"=0.0}, "Y Power Multiplier"=6.0, "Turn Power Multiplier"=5.0, "Gyro Output"=0.85, "Creep Rate"=0.4, "Distance Drive PID Gains"={"proportional gain (Kc)"=1.0, "integral time (Ti, min)"=0.01, "derivative time (Td, min)"=0.0}, "Distance Tolerance"=1.4999999999999998, "Distance Output"=0.85, "Strafe Threshold"=0.4, "Strafe Correct"=FALSE, "Strafe Tolerance"=0.0, "Translate Drive PID Gains"={"proportional gain (Kc)"=1.0, "integral time (Ti, min)"=0.01, "derivative time (Td, min)"=0.0}, "Strafe Output"=0.0, "SC Right"=0.85, "SC Left"=0.85, "Use Gyro"=FALSE, "Constant Power"=FALSE, "Strafe Power"=0.0, "Input Modifier"=enum."None", "SCR Delay"=0.85, "SCL Delay"=0.85}, "Intake Presets "={"Intake Speed "=0.0, "Outake Speed"=0.0, "Current Trip Delay"=0.0, "Max Current"=0.0, "Gear Outtake Motor Delay"=0.0, "Gear Intake Motor Delay"=0.0, "Gear Intake Pull Up Speed"=0.0, "Pusher Delay"=0.0, "Release Delay"=0.0, "Close Release Delay"=0.0}, "Shooter Presets"={"Key Shot"={"RPM "=0.0, "Hood?"=FALSE}, "Distance Shot"={"RPM"=0.0, "Hood?"=FALSE}, "RPM Tolerance"=0.0, "Unstuck Delay Time "=0.0, "Initial RPM Increase"=0.0, "Warmup Delay"=0.0, "Faster Time"=0.0, "Shooter PID Gains"={"P"=0.0, "I"=0.0, "D"=0.0, "FF"=0.0, "Ramp Rate"=0.0, "I Zone"=0.0}, "Unstuck Trigger Power"=0.0, "Trigger Power"=0.0, "Unstuck RPM"=0.0, "Agitator Active Power"=0.0, "Agitator Idle Power"=0.0, "RPM Tuning Range"=0.0, "RPM M Tuning Range"=0.0}, "Vision Target Packet"={"Robot Center"=0.0, "Center X"=0.0, "Center Y"=0.0, "Angle"=0.0, "Distance"=0.0, "Found Target?"=FALSE}, "Auton Presets"={"Start Position"=0.0}, "Drivetrain Encoder Values"={"Left Encoder"={"Distance"=0.0, "Speed"=0.0, "Tick"=0.0}, "Center Encoder"={"Distance"=0.0, "Speed"=0.0, "Tick"=0.0}, "Right Encoder"={"Distance"=0.0, "Speed"=0.0, "Tick"=0.0}}, "Drivetrain Encoder Settings"={"Left Tick Constant"=0.0, "Right Tick Contant"=0.0, "Reset Encoders"=FALSE, "Center Tick Constant"=0.0}, "Zero Gyro"=FALSE, "Vision Timeout"=0.0, "Pressure M"=0.0, "Pressure B"=0.0, "Auto Agitator"={"Enable Auto Agitation"=FALSE, "Continuous Stir"=FALSE, "Continuous Intake"=FALSE, "Alternate In/Outtake"=FALSE, "Wing Delay"=0.0, "Stir Delay"=0.0, "Intake Delay"=0.0, "Wing On Time"=0.0, "Wing Off Time"=0.0, "Stir On Time"=0.0, "Stir Off Time"=0.0, "Intake On Time"=0.0, "Intake Off Time"=0.0, "Stir Power"=0.0, "Intake Power"=0.0, "Outtake Power"=0.0, "Intake Run Time"=0.0, "Outtake Run Time"=0.0, "Wing$"=FALSE, "Intake"=FALSE, "Stirrer"=FALSE}, "Climber Settings"={"Climber Power"=0.0, "Max Current"=0.0, "Avoid Current Trip?"=FALSE}, "LEDs"={"Back"={"Default"="", "Traction"="", "Gear Ready Close"="", "Break On"="", "Gear Loaded"="", "Climb"="", "Gear Ready Far"="", "Unload Gear"="", "Prime Unload"=""}, "Front"={"Default"="", "Traction"="", "Gear Ready Close"="", "Break On"="", "Gear Loaded"="", "Climb"="", "Gear Ready Far"="", "Unload Gear"="", "Prime Unload"=""}, "LEDOnTime"=0.0, "LEDOffTime"=0.0}} ("Dashboard Packet"), "Drivetrain Settings"="Drivetrain Settings", "Drivetrain Encoder Settings"="Drivetrain Encoder Settings", "Intake Presets"="Intake Presets", "Shooter Presets"="Shooter Presets", "Auton Presets"="Auton Presets", "Zero Gyro"=w73, "Vision Timeout"="Vision Timeout", "Pressure M"="Pressure M", "Pressure B"="Pressure B", "Auto Agitator"="Auto Agitator", "Climber Settings"="Climber Settings", "LEDs"=w53) -> (w77:T51)
    n18 = Flatten To String(anything=w77) -> (data string=w78:string)  [unwired: 3 in, 2 out]
    n19 = local read "Robot IP"() -> (w79:string)
    n20 = Wait (ms)(milliseconds to wait=u32 1000) -> ()  [unwired: 1 out]
    n21 = call "DumbDash Send.vi"("Robot IP"=w79, "data string"=w78) -> ()  [unwired: 10 in]
  }
  n22 = register-events(refnum<vi> refnum, w20) -> (reference out=w18:refnum<event-registration>, error out=w17:errorcluster)  [unwired: 2 in]
  n23 = vi-ref "Playback Controls.vi"() -> (w16:refnum<vi>)
  n24 = property class="VI"() -> ("Panel"=w38:refnum<vi>)  [unwired: 2 in, 2 out]
  n25 = while {
    tunnel: w32 -> [w101]
    tunnel: w27 -> [w99]
    tunnel: [w97] -> _
    tunnel: u32 1000 ("milliseconds to wait") -> [w96]
    tunnel: w20 -> [w90]
    i -> [w97]
    stop <- FALSE stop-if-true
    n26 = local read "Rec Mode"() -> (w92:enum32{"Stop", "Record", "Playback"})
    n27 = Wait on Notification(notifier=w99, timeout in ms (-1)=w96) -> (notification=w98:string, timed out?=w94:bool)  [unwired: 2 in, 2 out]
    n28 = Equal?(x=w92, y=u16 2 ("Rec Mode")) -> (x = y?=w93:bool)
    n29 = Compound Arithmetic op=OR(invert w94, w93) -> (w95:bool)
    n30 = case shown="True" w95 {
      tunnel: w101 -> [_ w104]
      tunnel: w98 -> [_ w103]
      tunnel: w90 -> [_ w102]
      frame False {
      }
      frame True {
        n31 = call <vilib>:"Bind Controls to SmartDashboard.vi"("RPC ref"=w102, "Bound Control Refs"=w104, "Server IP Address"=w103) -> ()  [unwired: 9 in]
      }
    }
  }
  n32 = property class="Pnl"(reference=w38) -> ("Panes[]"=w39:refnum<vi>[])  [unwired: 1 in, 2 out]
  n33 = Index Array(array=w39) -> (element=w37:refnum<vi>)  [unwired: 1 in]
  n34 = call "624WPIAdjust Dashboard Window.vi"("Width"=1340, "Height"=500, "VI"=w15, "Notifier in"=w24) -> ()  [unwired: 8 in]
  n35 = while {
    tunnel: w37 -> [w106]
    i -> [w109]
    stop <- FALSE stop-if-true
    n36 = Wait (ms)(milliseconds to wait=u32 100) -> ()  [unwired: 1 out]
    n37 = case shown="\"Stop\", Default" "Rec Mode" {
      tunnel: w109 -> [_ _ w124]
      tunnel: [u32 2829099 ("Base Color") u32 11141120 ("Target Color") w113] -> w105
      frame "Stop", Default {
        # "Reset the color, extra updates don't cost much"
      }
      frame "Record" {
      }
      frame "Playback" {
        # "Playback"
        n38 = Quotient & Remainder(x=w124, y=u32 50 ("milliseconds to wait")) -> (x-y*floor(x/y)=w120:u32)  [unwired: 1 out]
        n39 = Divide(x=w120, y=u32 50 ("milliseconds to wait")) -> (x/y=w117:dbl)
        n40 = Multiply(x=6.283185307179586, y=w117) -> (x*y=w122:dbl)
        n41 = Sine(x=w122) -> (sin(x)=w121:dbl)
        n42 = Absolute Value(x=w121) -> (abs(x)=w114:dbl)
        n43 = call "Interpolate RGB Color.vi"("Proportion"=w114, "Target Color"=u32 30976, "Base Color"=u32 2829099) -> ("Result Color"=w113:u32)  [unwired: 8 in]
      }
    }
    n44 = property class="Pane"(reference=w106, "PaneColor"=w105) -> ()  [unwired: 1 in, 2 out]
  }
  n45 = call "IMAQ Create"("Image Name"="Gear Watcher", "Image Type"=w6) -> ("New Image"=w5:T2)  [unwired: 2 in, 2 out]
  n46 = call "IMAQ Create"("Image Name"="Goal Detection", "Image Type"=w46) -> ("New Image"=w44:T2)  [unwired: 2 in, 2 out]
  n47 = call "IMAQ Create"("Image Name"="Goal Mask", "Image Type"=w9) -> ("New Image"=w8:T2)  [unwired: 2 in, 2 out]
  n48 = call "IMAQ Create"("Image Name"="Gear Mask", "Image Type"=w3) -> ("New Image"=w1:T2)  [unwired: 2 in, 2 out]
  n49 = while {
    tunnel: w5 -> [w129]
    tunnel: w1 -> [_]
    stop <- FALSE stop-if-true
    n50 = local read "Rec Mode"() -> (w131:enum32{"Stop", "Record", "Playback"})
    n51 = Wait (ms)(milliseconds to wait=u32 1) -> ()  [unwired: 1 out]
    n52 = call "624WPI_CameraRead MJPG for Dashboard.vi"("Recording Name"="Axis", "Camera Settings"="Gear Camera Settings", "Rec Mode"=w131, "Camera IP"="axis-camera2.local", "Camera Mode"="Camera Mode 2", "Refnum in"=w129) -> ("Active"=w134:bool, "Refnum out"=w125:T2, "FPS"=w136:dbl, "Bandwidth (Mbps)"=w135:dbl)  [unwired: 2 in]
    n53 = case shown="True" w134 {
      tunnel: w125 -> [_ _]
      tunnel: w136 -> [_ w203]
      tunnel: w135 -> [_ w202]
      tunnel: w125 -> [_ w172]
      frame False {
      }
      frame True {
        w176 = u16 2 items=["RGB", "HSL", "HSV", "HSI"] ("Color Mode")
        w185 = u16 2 items=["RGB", "HSL", "HSV", "HSI", "CIE L*a*b*", "CIE XYZ"] ("Color Mode")
        w198 = 0.04  # Size Limit %
        # "Update Mbps LED"
        n54 = case shown="4, 5" w202 {
          tunnel: [u32 6618880 ("Color Box") u32 16776722 ("Color Box") u32 16716800 ("Color Box")] -> w207
          frame Default {
          }
          frame 4, 5 {
          }
          frame 6.. {
          }
        }
        n55 = local read "Gear LED Color"() -> (w177:T3)
        n56 = Bundle("Color Box"=w207, "Color Box"=w207) -> (w208:cluster{"Color Box":u32, "Color Box":u32})  [unwired: 1 out]
        n57 = Bundle(FALSE, "Bandwidth (Mbps)"=w202, "FPS"=w203) -> (→"Camera Info 3":cluster{bool, "Bandwidth (Mbps)":dbl, "FPS":dbl})  [unwired: 1 in]
        n58 = Build Array(w208) -> (w206:cluster{"Color Box":u32, "Color Box":u32}[])
        n59 = call "IMAQ Clear Overlay"("Image"=w172) -> ("Image Out"=w137:T2)  [unwired: 9 in, 1 out]
        "Gear Original Image" <- w137
        "Gear Cam" <- w137
        n60 = property on="Mbps LED" class="Bool (strict)"("Colors [4]"=w206) -> ()  [unwired: 2 in, 2 out]
        n61 = control-ref of="Gear Original Image"() -> (w184:refnum<vi>)
        n62 = First Call?() -> (First Call?: T/F=w183:bool)
        n63 = Not(x=w183) -> (.not. x?=w181:bool)
        n64 = call "Calibration Helper2.vi"("Color Mode"=w185, "Color Components"=w177, "Image"=w137, "Image Ctl Refnum"=w184) -> ("Changed"=w182:bool, "output color"=w179:T53)  [unwired: 6 in]
        n65 = And(x=w182, y=w181) -> (x .and. y?=w178:bool)
        n66 = case shown="True" w178 {
          tunnel: w179 -> [_ w209]
          frame False {
          }
          frame True {
            n67 = local write "Gear LED Color"(w209) -> ()
          }
        }
        n68 = Select(t=w179, s=w178, f=w177) -> (s? t:f=w180:T3)
        n69 = Unbundle(w180) -> ("Hue"=w199:cluster{dbl, dbl}, "Sat"=w200:cluster{dbl, dbl}, "Val"=w201:cluster{dbl, dbl})
        n70 = call "IMAQ ColorThreshold"("Blue or Luma or Val or Inten Range"=w201, "Replace Value"=1, "Green or Sat Range"=w200, "Color Mode"=w176, "Red or Hue Range"=w199, "Image Src"=w137) -> ("Image Dst Out"=w174:T2)  [unwired: 4 in, 1 out]
        "Gear Masked Image" <- w174
        n71 = call "Sorted Particle Report 2016.vi"("Min Area Size %"=w198, "Particle Count Limit"="Particles 2", "Image in"=w174) -> ("Sorted Data"=w196:dbl[][], "Particles"=→"Gear Qualified Particles":i32)  [unwired: 1 in]
        n72 = call "Cull and Group.vi"("Line Border"="Line Border 2", "Score Cutoff"="Gear Score Cutoff %", "Sorted Data"=w196) -> ("Rect"=w189:T54, "Line"=w186:T54, "Score"=w190:dbl, "Center"=w191:cluster{"X":dbl, "Y":dbl})  [unwired: 5 in]
        n73 = call "Compute DistanceToTarget2.vi"("Calibrated"="Gear Use Calibration", "Camera Type"="Gear Camera Type", "Line"=w186, "Image Src"=w137) -> ("Distance (ft)"=w192:dbl, "Image Dst Out"=w188:T2)  [unwired: 5 in, 1 out]
        n74 = call "Normalize Coordinates.vi"("Score"=w190, "Center"=w191, "Distance"=w192, "Bounding box"=w189, "Image in"=w188) -> ("Results"=w171:T32)  [unwired: 5 in, 1 out]
        "Gear Results" <- w171
        n75 = Unbundle By Name(w171) -> ("Distance (ft)"=w140:dbl, "Normalized.Center"=w147:cluster{dbl, dbl}, "Normalized.Rectangle"=w141:T55)
        n76 = Not Equal?(x=w140, y=inf) -> (x != y?=w138:bool)
        n77 = call "IMAQ GetImageSize"("Image"=w137) -> ("Y Resolution"=w153:i32, "X Resolution"=w145:i32)  [unwired: 3 in, 1 out]
        n78 = Unbundle(w147) -> (w146:dbl)  [unwired: 1 out]
        n79 = Divide(x=w145, y=2) -> (x/y=w150:dbl)
        n80 = call "Gear Calculate Angle.vi"("Normalized.Rectangle"=w141, "Goal Display"=w137) -> ("Angle Difference"=w142:dbl)  [unwired: 9 in]
        n81 = Multiply(x=w150, y=w146) -> (x*y=w159:dbl)
        n82 = Add(x=w159, y=w150) -> (x+y=w154:dbl)
        n83 = Bundle By Name(cluster="Gear Vision Packet 2", "Distance"=w140, "Angle"=w142, "Found Target?"=w138) -> (→"Gear Vision Packet":T1)
        n84 = Bundle(cluster=cluster{"X":i32, "Y":i32} {"X"=0, "Y"=0} ("Start Point"), "X"=w154, "Y"=0) -> (w156:cluster{"X":i32, "Y":i32})
        n85 = Bundle(cluster=cluster{"X":i32, "Y":i32} {"X"=0, "Y"=0} ("Start Point"), "X"=w154, "Y"=w153) -> (w152:cluster{"X":i32, "Y":i32})
        n86 = call <vilib>:"Get Translation.vi"() -> ()  [unwired: 9 in, 3 out]
        n87 = call "IMAQ Overlay Line"("Color"=u32 16711680, "End Point"=w152, "Start Point"=w156, "Image"=w137) -> ("Image Out"=w149:T2)  [unwired: 6 in, 1 out]
        n88 = call "IMAQ GetImageSize"("Image"=w149) -> ("Y Resolution"=w163:i32, "X Resolution"=w170:i32)  [unwired: 3 in, 1 out]
        n89 = Divide(x=w170, y=2) -> (x/y=w164:dbl)
        n90 = Bundle By Name(cluster=cluster{"X":i32, "Y":i32} {"X"=0, "Y"=0} ("Start Point"), "X"=w164, "Y"=0) -> (w167:cluster{"X":i32, "Y":i32})
        n91 = Bundle By Name(cluster=cluster{"X":i32, "Y":i32} {"X"=0, "Y"=0} ("End Point"), "X"=w164, "Y"=w163) -> (w162:cluster{"X":i32, "Y":i32})
        n92 = call "IMAQ Overlay Line"("Color"=u32 6618880, "End Point"=w162, "Start Point"=w167, "Image"=w149) -> ("Image Out"=→"Gear Front Cam":T2)  [unwired: 6 in, 1 out]
        n93 = call <vilib>:"Set Translation.vi"() -> ()  [unwired: 10 in, 2 out]
      }
    }
  }
  n94 = call <vilib>:"Intialize Keyboard.vi"() -> ("device ID"=w4:refnum<k1>)  [unwired: 10 in, 1 out]
  n95 = while {
    tunnel: w44 -> [w220]
    tunnel: [w225] -> _
    tunnel: w21 -> [w218]
    tunnel: w8 -> [w215]
    i -> [w225]
    stop <- FALSE stop-if-true
    n96 = local read "Rec Mode"() -> (w214:enum32{"Stop", "Record", "Playback"})
    n97 = call "624WPI_CameraRead MJPG for Dashboard.vi"("Recording Name"="Axis2", "Camera Settings"="Camera Settings", "Rec Mode"=w214, "Camera IP"="axis-camera.local", "Camera Mode"="Camera Mode", "Refnum in"=w220) -> ("Active"=w217:bool, "Refnum out"=w223:T2, "FPS"=w222:dbl, "Bandwidth (Mbps)"=w221:dbl)  [unwired: 2 in]
    n98 = case shown="True" w217 {
      tunnel: w223 -> [w227 w290]
      tunnel: w221 -> [_ w286]
      tunnel: w222 -> [_ w285]
      tunnel: w218 -> [_ w291]
      tunnel: w217 -> [_ _]
      tunnel: [w227 _] -> _
      tunnel: w215 -> [_ w262]
      frame False {
        w229 = u32 1985280 ("Color Box")
        # "Sleep for 500ms"
        n99 = Bundle("Color Box"=w229, "Color Box"=w229) -> (w230:cluster{"Color Box":u32, "Color Box":u32})  [unwired: 1 out]
        n100 = Build Array(w230) -> (w228:cluster{"Color Box":u32, "Color Box":u32}[])
        n101 = property on="Mbps LED" class="Bool (strict)"("Colors [4]"=w228) -> ()  [unwired: 2 in, 2 out]
        n102 = Wait Until Next ms Multiple(millisecond multiple=u32 500) -> ()  [unwired: 1 out]
      }
      frame True {
        w276 = u16 2 items=["RGB", "HSL", "HSV", "HSI"] ("Color Mode")
        w289 = u16 2 items=["RGB", "HSL", "HSV", "HSI", "CIE L*a*b*", "CIE XYZ"] ("Color Mode")
        w304 = 0.04  # Size Limit %
        # "Read from Camera"
        # "Update Mbps LED"
        n103 = local read "LED Color"() -> (w277:T3)
        n104 = case shown="4, 5" w286 {
          tunnel: [u32 6618880 ("Color Box") u32 16776722 ("Color Box") u32 16716800 ("Color Box")] -> w310
          frame Default {
          }
          frame 4, 5 {
          }
          frame 6.. {
          }
        }
        n105 = control-ref of="Original Image"() -> (w284:refnum<vi>)
        n106 = call "IMAQ Clear Overlay"("Image"=w290) -> ("Image Out"=w245:T2)  [unwired: 9 in, 1 out]
        "Original Image" <- w245
        n107 = Bundle("Color Box"=w310, "Color Box"=w310) -> (w311:cluster{"Color Box":u32, "Color Box":u32})  [unwired: 1 out]
        n108 = Bundle(FALSE, "Bandwidth (Mbps)"=w286, "FPS"=w285) -> (→"Camera Info":cluster{bool, "Bandwidth (Mbps)":dbl, "FPS":dbl})  [unwired: 1 in]
        n109 = First Call?() -> (First Call?: T/F=w283:bool)
        n110 = Build Array(w311) -> (w309:cluster{"Color Box":u32, "Color Box":u32}[])
        n111 = Not(x=w283) -> (.not. x?=w281:bool)
        n112 = call "Calibration Helper2.vi"("Color Mode"=w289, "Color Components"=w277, "Image"=w245, "Image Ctl Refnum"=w284) -> ("Changed"=w282:bool, "output color"=w279:T53)  [unwired: 6 in]
        n113 = property on="Mbps LED" class="Bool (strict)"("Colors [4]"=w309) -> ()  [unwired: 2 in, 2 out]
        n114 = And(x=w282, y=w281) -> (x .and. y?=w278:bool)
        n115 = Select(t=w279, s=w278, f=w277) -> (s? t:f=w280:T3)
        n116 = case shown="True" w278 {
          tunnel: w279 -> [_ w320]
          frame False {
          }
          frame True {
            n117 = local write "LED Color"(w320) -> ()
          }
        }
        n118 = Unbundle(w280) -> ("Hue"=w305:cluster{dbl, dbl}, "Sat"=w306:cluster{dbl, dbl}, "Val"=w307:cluster{dbl, dbl})
        n119 = call "IMAQ ColorThreshold"("Blue or Luma or Val or Inten Range"=w307, "Replace Value"=1, "Green or Sat Range"=w306, "Color Mode"=w276, "Red or Hue Range"=w305, "Image Dst"=w262, "Image Src"=w245) -> ("Image Dst Out"=w274:T2)  [unwired: 3 in, 1 out]
        "Masked Image" <- w274
        n120 = call "Sorted Particle Report 2016.vi"("Min Area Size %"=w304, "Particle Count Limit"="Particles", "Pixel Measurements"=w291, "Image in"=w274) -> ("Sorted Data"=w302:dbl[][], "Particles"=→"Qualified Particles":i32)
        n121 = call "Cull and Group.vi"("Line Border"="Line Border", "Score Cutoff"="Score Cutoff %", "Sorted Data"=w302) -> ("Rect"=w295:T54, "Line"=w292:T54, "Score"=w296:dbl, "Center"=w297:cluster{"X":dbl, "Y":dbl})  [unwired: 5 in]
        n122 = call "Compute DistanceToTarget2.vi"("Calibrated"="Use Calibration", "Camera Type"="Camera Type", "Line"=w292, "Image Src"=w245) -> ("Distance (ft)"=w298:dbl, "Image Dst Out"=w294:T2)  [unwired: 5 in, 1 out]
        n123 = call "Normalize Coordinates.vi"("Score"=w296, "Center"=w297, "Distance"=w298, "Bounding box"=w295, "Image in"=w294) -> ("Results"=w261:T32)  [unwired: 5 in, 1 out]
        "Results" <- w261
        n124 = Unbundle By Name(w261) -> ("Normalized.Rectangle"=w244:T55, "Normalized.Center"=w258:cluster{dbl, dbl}, "Distance (ft)"=w234:dbl)
        "Distance from Target" <- w234
        n125 = call "IMAQ GetImageSize"("Image"=w245) -> ("Y Resolution"=w251:i32, "X Resolution"=w260:i32)  [unwired: 3 in, 1 out]
        n126 = call "Calculate Angle.vi"("Normalized.Rectangle"=w244, "Goal Display"=w245) -> ("Angle Difference"=w233:dbl)  [unwired: 9 in]
        "Target Angle Difference" <- w233
        n127 = Unbundle(w258) -> (w247:dbl)  [unwired: 1 out]
        n128 = Divide(x=w260, y=2) -> (x/y=w246:dbl)
        n129 = Not Equal?(x=w234, y=inf) -> (x != y?=w232:bool)
        "Target Found?" <- w232
        n130 = Multiply(x=w246, y=w247) -> (x*y=w257:dbl)
        n131 = Bundle By Name(cluster=T33 {"Distance"=0.0, "Angle"=0.0, "Found Target?"=FALSE} ("Goal Vision Packet"), "Distance"=w234, "Angle"=w233, "Found Target?"=w232) -> (w239:T33)
        "Goal Vision Packet" <- w239
        n132 = Add(x=w257, y=w246) -> (x+y=w252:dbl)
        n133 = Bundle(cluster=cluster{"X":i32, "Y":i32} {"X"=0, "Y"=0} ("Start Point"), "X"=w252, "Y"=0) -> (w254:cluster{"X":i32, "Y":i32})
        n134 = Bundle(cluster=cluster{"X":i32, "Y":i32} {"X"=0, "Y"=0} ("Start Point"), "X"=w252, "Y"=w251) -> (w250:cluster{"X":i32, "Y":i32})
        n135 = local read "Robot IP"() -> (w241:string)
        n136 = Flatten To String(anything=w239) -> (data string=w238:string)  [unwired: 3 in, 2 out]
        n137 = call "IMAQ Overlay Line"("Color"=u32 16711680, "End Point"=w250, "Start Point"=w254, "Image"=w245) -> ("Image Out"=w248:T2)  [unwired: 6 in, 1 out]
        n138 = call "IMAQ GetImageSize"("Image"=w248) -> ("Y Resolution"=w266:i32, "X Resolution"=w273:i32)  [unwired: 3 in, 1 out]
        n139 = Divide(x=w273, y=2) -> (x/y=w267:dbl)
        n140 = Bundle By Name(cluster=cluster{"X":i32, "Y":i32} {"X"=0, "Y"=0} ("Start Point"), "X"=w267, "Y"=0) -> (w270:cluster{"X":i32, "Y":i32})
        n141 = Bundle By Name(cluster=cluster{"X":i32, "Y":i32} {"X"=0, "Y"=0} ("End Point"), "X"=w267, "Y"=w266) -> (w265:cluster{"X":i32, "Y":i32})
        n142 = call "IMAQ Overlay Line"("Color"=u32 6618880, "End Point"=w265, "Start Point"=w270, "Image"=w248) -> ("Image Out"=→"Front Camera Display":T2)  [unwired: 6 in, 1 out]
        n143 = First Call?() -> (First Call?: T/F=w237:bool)
        n144 = Empty String/Path?(string/path=w241) -> (empty?=w240:bool)
        n145 = feedback #1() -> (w236:refnum<k16>)  [unwired: 1 in]
        n146 = case shown="False" w237 {
          tunnel: [w312 w313] -> w235
          tunnel: w236 -> [w312 _]
          frame False {
          }
          frame True {
            n147 = UDP Open(11:u16 0 ("port")) -> (port=w313:refnum<k16>)  [unwired: 4 in, 2 out]
          }
        }
        n148 = case shown="True" w240 {
          tunnel: w241 -> [w317 _]
          tunnel: w238 -> [w319 _]
          tunnel: w235 -> [w315 _]
          frame False {
            n149 = String To IP(1:w317) -> (0:w316:u32)
            n150 = UDP Write(address=w316, port or service name=u16 5805, connection ID=w315, data in=w319) -> ()  [unwired: 2 in, 2 out]
          }
          frame True {
          }
        }
        n151 = feedback-in #1(w235) -> ()
      }
    }
  }
  n152 = while {
    tunnel: w4 -> [w329]
    stop <- FALSE stop-if-true
    n153 = call-poly <vilib>:"Acquire Input Data.vi"("device ID"=w329) -> ("keys pressed"=w327:T57)  [unwired: 16 in, 2 out]
    n154 = case shown="True" "Open in Excel" {
      frame False {
      }
      frame True {
        n155 = flat-sequence {
          frame #0 {
            n156 = invoke on="Shooter RPM History" class="WFChart (strict)" method="Export Data to Excel"() -> ()  [unwired: 3 in, 3 out]
          }
          frame #1 {
            n157 = local write "Open in Excel"(FALSE ("Open in Excel")) -> ()
          }
        }
      }
    }
    n158 = Search 1D Array(1D array=w327, element=T56."G") -> (index of element=w326:i32)  [unwired: 1 in]
    n159 = Greater Or Equal To 0?(x=w326) -> (x >= 0?=w325:bool)
    n160 = local write "Zero Gyro"(w325) -> ()
    n161 = Wait (ms)(milliseconds to wait=u32 1) -> ()  [unwired: 1 out]
  }
  n162 = while {
    tunnel: u16 1741 ("timeout ms (25000)") -> [w334]
    stop <- FALSE stop-if-true
    n163 = TCP Create Listener(10:w334) -> (0:w333:errorcluster, 3:w335:refnum<k5>)  [unwired: 4 in, 1 out]
    n164 = case shown="No Error" w333 {
      selector: w333 -> [w337 _]
      tunnel: w335 -> [w338 _]
      frame No Error {
        n165 = while {
          tunnel: w338 -> [w341]
          tunnel: w337 -> [w340]
          stop <- FALSE stop-if-true
          n166 = TCP Wait On Listener(8:w340, 11:w341) -> (0:w342:errorcluster, 4:w343:refnum<k5>)  [unwired: 2 in, 3 out]
          n167 = local write "TCP"(w343) -> ()
          n168 = case shown="No Error" w342 {
            frame No Error {
            }
            frame Error {
              n169 = Wait (ms)(milliseconds to wait=u32 1000) -> ()  [unwired: 1 out]
            }
          }
        }
      }
      frame Error {
        n170 = Wait (ms)(milliseconds to wait=u32 1000) -> ()  [unwired: 1 out]
      }
    }
  }
  n171 = while {
    tunnel: [w346] -> _
    tunnel: w27 -> [w355]
    tunnel: w24 -> [w356]
    i -> [w346]
    stop <- FALSE stop-if-true
    n172 = call "624WPI_DashboardGetInfo.vi"("Binding Refnum"=w355, "Window Mode Notifier"=w356, "TCP Cnx"="TCP") -> ("Power and Errors"=w351:T5, "Robot Metrics"=w352:T45, "Status Info"=w353:T43, "Control Info"=w354:T44, "Robot Mode"=w350:T63, "Process?"=w348:bool, "Custom Dashboard Data"=w349:string)  [unwired: 2 in]
    n173 = Wait (ms)(milliseconds to wait=u32 4) -> ()  [unwired: 1 out]
    n174 = case shown="True" w348 {
      tunnel: w353 -> [_ w535]
      tunnel: w352 -> [_ w534]
      tunnel: w354 -> [_ w536]
      tunnel: w351 -> [_ w533]
      tunnel: w350 -> [_ _]
      tunnel: w349 -> [_ w539]
      tunnel: w346 -> [_ w413]
      frame False {
        n175 = Wait (ms)(milliseconds to wait=u32 20) -> ()  [unwired: 1 out]
      }
      frame True {
        w464 = "\\" ("string")
        n176 = Unbundle By Name(w533) -> ("Robot IP"=→"Robot IP":string)
        n177 = Unflatten From String(type=T58 {"Climb Status Cluster"={"Climb Speed"=0.0}, "Drivetrain Status Cluster"={"Y (Throttle)"=0.0, "X (Steer)"=0.0, "Z (Strafe)"=0.0, "Heading Target"=0.0, "Center Piston Down?"=FALSE, "Traction?"=FALSE, "Gyro Steer Finished?"=FALSE, "Distance Drive Finished?"=FALSE, "Gyro"=0.0, "Distance Target"=0.0, "Y Max Output"=0.0, "Y Min Output"=0.0, "X Max Output"=0.0, "X Min Output"=0.0, "Z Max Output"=0.0, "Z Min Output"=0.0, "Translation Target"=0.0, "Translation Drive Finished?"=FALSE, "PID Auto Drive Finished?"=FALSE, "Brake?"=FALSE, "Vision Aligned?"=FALSE, "Creep Mode Engaged?"=FALSE, "Drivetrain Mode"=enum."Manual", "Gear Vision Aligned?"=FALSE}, "Intake Status Cluster"={"Roller Power"=0.0, "Intake Mode"=enum."Manual", "Intake Auto State"=enum."Idle", "Backward Tripped?"=FALSE, "Forward Tripped?"=FALSE, "Intake Current Trip State"=enum."Normal", "Gear Flap Open"=FALSE, "Doors Open"=FALSE, "Traction for Gear?"=FALSE, "Current"=0.0, "Intake Down?"=FALSE, "Gear Loaded"=FALSE, "Pusher Activated"=FALSE, "Gear Load State"=enum."Idle", "Unload Mode"=enum."None", "Unloading Gear?"=FALSE}, "Shooter Status Cluster"={"Current RPM"=0.0, "Trigger Power"=0.0, "Shooter Mode"=enum."Auto", "Shot Type"=enum."Dist Shot", "Shooter State"=enum."Idle ", "Target RPM"=0.0, "Hood Down?"=FALSE, "RPM Reached?"=FALSE, "User Inputed RPM"=0.0}, "Drivetrain Encoder Values"={"Left Encoder"={"Distance"=0.0, "Speed"=0.0, "Tick"=0.0}, "Center Encoder"={"Distance"=0.0, "Speed"=0.0, "Tick"=0.0}, "Right Encoder"={"Distance"=0.0, "Speed"=0.0, "Tick"=0.0}}, "Auton Command Cluster"={"commandID"=0.0, "maxTime"=0.0, "distanceTarget"=0.0, "headingTarget"=0.0, "translationTarget"=0.0, "ySpeed"=0.0, "xSpeed"=0.0, "zSpeed"=0.0, "async"=0.0, "shotType"=0.0, "shootCommand"=0.0, "rollerPower"=0.0, "fillHopper?"=0.0, "zeroGyro"=0.0, "openGear"=0.0, "traction?"=0.0}, "Auton File Lists"={"Current Queue"="", "General Scripts"="", "Movements"=""}, "Pressure"=0.0, "Pressure Voltage"=0.0, "Motor Operational Status"={"Sensor Velocity "=0.0, "Encoder Position"=0.0, "Encoder Velocity "=0.0, "Encoder Index Count"=0.0, "Analog In"=0.0, "Analog In Velocity"=0.0, "Battery Voltage"=0.0, "Current"=0.0, "Sensor Position"=0.0, "Vel Div 4"=FALSE, "Encoder A Pin State"=FALSE, "Encoder B Pin State"=FALSE, "Encoder Index Pin State"=FALSE, "Pulse Width Velocity "=0.0}, "Vision Presets"=[], "Climber Current Tripped?"=FALSE, "Gear?"=FALSE, "PDP Status Cluster"={"Drivetrain Left CIM 1"=0.0, "Drivetrain Left CIM 2"=0.0, "Drivetrain Left Mini CIM"=0.0, "Drivetrain Right CIM 1"=0.0, "Drivetrain Right CIM 2"=0.0, "Drivetrain Right Mini CIM"=0.0, "Drivetrain Center CIM 1"=0.0, "Drivetrain Center CIM 2"=0.0, "Shooter Motor 1"=0.0, "Shooter Motor 2"=0.0, "Climber Motor 1"=0.0, "Climber Motor 2"=0.0, "Intake Motor"=0.0, "Trigger Motor"=0.0, "Fans/Compressor"=0.0}, "Robot Status Cluster"={"RobotMode"=enum."Autonomous Disabled", "Alliance"=enum."Red", "Position"=enum."1", "Match Time"=0.0, "FMS?"=FALSE}, "LED Status Cluster"={"Front Red"=FALSE, "Front Green"=FALSE, "Front Blue"=FALSE, "Back Red"=FALSE, "Back Green"=FALSE, "Back Blue"=FALSE}, "PIXY Vision Packet"={"Objects"=[]}} ("Dashboard Status Data"), binary string=w539) -> (value=w537:T58)  [unwired: 3 in, 2 out]
        n178 = Unbundle By Name(w537) -> ("Drivetrain Status Cluster"=w528:T16, "Intake Status Cluster"=w363:T18, "Shooter Status Cluster"=w360:T23, "Drivetrain Encoder Values"=w501:T14, "Auton Command Cluster"=→"Auton Command Cluster":T35, "Auton File Lists"=w449:T34, "Pressure"=→"Pressure" →"Pressure":dbl, "Pressure Voltage"=→"Pressure Voltage":dbl, "Motor Operational Status"=→"Motor Operational Status":T26, "Vision Presets"=→"Distance Shots":T29, "Climber Current Tripped?"=→"Climber Current Tripped" →"Climber Tripped":bool, "PDP Status Cluster"=w452:T60, "Robot Status Cluster"=w447:T37, "Climb Status Cluster.Climb Speed"=→"Climber Power":dbl, "LED Status Cluster"=w371:T61)
        "Drivetrain Encoder Values" <- w501
        "Drivetrain Status Cluster" <- w528
        "Auton File Lists" <- w449
        "PDP Currents" <- w452
        "Robot Status Cluster" <- w447
        "Shooter Status Cluster" <- w360
        "Intake Status Cluster" <- w363
        n179 = local read "Goal Vision Packet"() -> (w518:T33)
        n180 = Cluster To Array(cluster=w452) -> (array=w451:dbl[])
        n181 = Add Array Elements(numeric array=w451) -> (sum=→"Total Current":dbl)
        n182 = local read "Rec Mode"() -> (w411:enum32{"Stop", "Record", "Playback"})
        n183 = local read "Rec Mode"() -> (w406:enum32{"Stop", "Record", "Playback"})
        n184 = Unbundle By Name(w528) -> ("Gyro"=w517:dbl, "Center Piston Down?"=w454:bool, "Traction?"=w459:bool, "Brake?"=→"Brakes":bool, "Vision Aligned?"=→"Vision Aligned?":bool, "Creep Mode Engaged?"=→"Creep Mode?":bool)
        "Center Wheel" <- w454
        "Traction" <- w459
        n185 = Unbundle By Name(w363) -> ("Gear Loaded"=→"Gear?":bool, "Gear Flap Open"=w431:bool, "Doors Open"=w439:bool, "Intake Auto State"=→"Intake State":T9, "Intake Mode"=w438:T19, "Backward Tripped?"=→"Backward Tripped?":bool, "Forward Tripped?"=→"Forward Tripped?":bool, "Roller Power"=→"Intake Power":dbl, "Intake Down?"=w463:bool, "Doors Open"=→"Doors Open?":bool, "Pusher Activated"=→"Pusher Activated?":bool)
        "Wings" <- w439
        "Gear" <- w431
        n186 = Unbundle By Name(w360) -> ("Target RPM"=w437:dbl, "Trigger Power"=→"Trigger Power":dbl, "Current RPM"=w453:dbl, "Shot Type"=→"Shot Type":T8, "Shooter State"=→"Shooter State":T7, "Shooter Mode"=w495:T24, "Hood Down?"=w469:bool, "RPM Reached?"=w490:bool)
        "Hood Down?" <- w469
        "Target RPM" <- w437
        "Current RPM" <- w453
        "Shooter RPM History" <- w453
        n187 = Unbundle By Name(w501) -> ("Left Encoder.Speed"=→"Left":dbl, "Right Encoder.Speed"=→"Right":dbl, "Center Encoder.Speed"=→"Center":dbl)
        n188 = Unbundle By Name(w449) -> ("Current Queue"=→"Current Auto Queue":string)
        n189 = Unbundle By Name(w447) -> ("Match Time"=w414:dbl, "RobotMode"=w402:T38)
        "Match Time\n(seconds)" <- w414
        n190 = Unbundle By Name(w518) -> ("Angle"=w516:dbl)
        n191 = Equal?(x=w411, y=enum32{"Stop", "Record", "Playback"}."Stop") -> (x = y?=w409:bool)
        n192 = Equal?(x=w406, y=enum32{"Stop", "Record", "Playback"}."Record") -> (x = y?=w404:bool)
        n193 = Negate(x=w517) -> (-x=w522:dbl)
        n194 = Equal?(x=w402, y=WPI_DriverStationRobotMode2."Autonomous Enabled" ("RobotMode")) -> (x = y?=w412:bool)
        n195 = Equal?(x=w402, y=WPI_DriverStationRobotMode2."Teleop Disabled" ("RobotMode")) -> (x = y?=w401:bool)
        n196 = Subtract(x=w517, y=w516) -> (x-y=w511:dbl)
        n197 = Less Or Equal?(x=w414, y=30.0) -> (x <= y?=w444:bool)
        n198 = Less Or Equal?(x=w414, y=10.0) -> (x <= y?=w443:bool)
        n199 = Absolute Value(x=w522) -> (abs(x)=w531:dbl)
        n200 = Less Or Equal To 0?(x=w522) -> (x <= 0?=w532:bool)
        n201 = To Time Stamp(1:w414) -> (0:w428:timestamp)
        n202 = case shown="False" w412 {
          tunnel: w444 -> [w547 _]
          tunnel: w443 -> [w546 _]
          tunnel: [w545 u32 16776770 ("Color")] -> w442
          tunnel: w414 -> [w544 _]
          tunnel: w413 -> [w543 _]
          frame False {
            n203 = case shown="True" w547 {
              tunnel: w546 -> [_ w552]
              tunnel: [u32 12369084 ("Color") w553] -> w545
              tunnel: w544 -> [_ _]
              tunnel: w543 -> [_ w556]
              frame False {
              }
              frame True {
                n204 = Select(t=25.0, s=w552, f=85.0) -> (s? t:f=w549:dbl)
                n205 = Select(t=u32 16711680 ("Color"), s=w552, f=u32 16776770 ("Color")) -> (s? t:f=w555:u32)
                n206 = Quotient & Remainder(x=w556, y=w549) -> (x-y*floor(x/y)=w559:dbl)  [unwired: 1 out]
                n207 = Divide(x=w559, y=w549) -> (x/y=w558:dbl)
                n208 = Multiply(x=6.283185307179586, y=w558) -> (x*y=w561:dbl)
                n209 = Sine(x=w561) -> (sin(x)=w560:dbl)
                n210 = Absolute Value(x=w560) -> (abs(x)=w557:dbl)
                n211 = call "Interpolate RGB Color.vi"("Proportion"=w557, "Target Color"=w555, "Base Color"=u32 12369084 ("Color")) -> ("Result Color"=w553:u32)  [unwired: 8 in]
              }
            }
          }
          frame True {
          }
        }
        n212 = Subtract(x=360.0, y=w531) -> (x-y=w529:dbl)
        n213 = Negate(x=w511) -> (-x=w515:dbl)
        n214 = Seconds To Date/Time(time stamp (now)=w428) -> (date time rec=w427:T64)  [unwired: 1 in]
        n215 = Select(t=w529, s=w532, f=w522) -> (s? t:f=w519:dbl)
        n216 = call-poly "Change Detect.vi"("In"=w402) -> ("Changed?"=w405:bool)
        n217 = Unbundle By Name(w427) -> ("minute"=w426:i32, "second"=w422:i32)
        n218 = Not Equal To 0?(x=w437) -> (x != 0?=w488:bool)
        n219 = Compound Arithmetic op=AND(w405, w412, w409) -> (w408:bool)
        n220 = Compound Arithmetic op=AND(w405, w401, w404) -> (w400:bool)
        n221 = case shown="True" w408 {
          frame False {
          }
          frame True {
            w542 = enum32{"Stop", "Record", "Playback"}."Record" ("Rec Mode")
            n222 = local write "Rec Mode"(w542) -> ()
            n223 = global write "WPI_DashboardLogging Global.vi" "Recording"(w542) -> ()
          }
        }
        n224 = case shown="True" w400 {
          frame False {
          }
          frame True {
            w541 = enum32{"Stop", "Record", "Playback"}."Stop" ("Rec Mode")
            n225 = local write "Rec Mode"(w541) -> ()
            n226 = global write "WPI_DashboardLogging Global.vi" "Recording"(w541) -> ()
          }
        }
        n227 = Absolute Value(x=w515) -> (abs(x)=w513:dbl)
        n228 = Equal?(x=w495, y=Shooter_Modes."Auto" ("Shooter Mode")) -> (x = y?=→"Shooter":bool)
        n229 = Equal?(x=w438, y=Intake_Modes."Auto" ("Intake Mode")) -> (x = y?=→"Intake":bool)
        n230 = Bundle(cluster=cluster{dbl, dbl} {0.0, 991.7530055329754} ("RPM"), w453, w437) -> (→"RPM":cluster{dbl, dbl})
        n231 = And(x=w488, y=w490) -> (x .and. y?=→"RPM Reached?":bool)
        n232 = Less Or Equal To 0?(x=w515) -> (x <= 0?=w512:bool)
        n233 = Subtract(x=360.0, y=w513) -> (x-y=w514:dbl)
        n234 = And(x=w459, y=w431) -> (x .and. y?=→"Complete Gear Load":bool)
        n235 = Select(t=w514, s=w512, f=w515) -> (s? t:f=w509:dbl)
        n236 = Bundle(cluster=cluster{dbl, dbl} {0.0, 147.13378677278754} ("Gyro"), w519, w509) -> (→"Gyro":cluster{dbl, dbl})
        n237 = Absolute Value(x=w422) -> (abs(x)=w421:i32)
        n238 = Less?(x=w421, y=10) -> (x < y?=w417:bool)
        n239 = Number To Decimal String(number=w426) -> (decimal integer string=w424:string)  [unwired: 1 in]
        n240 = Number To Decimal String(number=w422) -> (decimal integer string=w416:string)  [unwired: 1 in]
        n241 = Or(x=w431, y=w463) -> (x .or. y?=w462:bool)
        n242 = Concatenate Strings("0" ("string"), w416) -> (w418:string)
        n243 = property on="Match Time" class="Str"("Text.BGColor"=w442, "Text.FG Color"=w442) -> ()  [unwired: 2 in, 2 out]
        n244 = Select(t=w418, s=w417, f=w416) -> (s? t:f=w415:string)
        n245 = Concatenate Strings(w424, ":" ("string"), w415) -> (→"Match Time":string)
        n246 = Unbundle By Name(w371) -> ("Front Red"=w370:bool, "Front Green"=w369:bool, "Front Blue"=w368:bool, "Back Red"=w367:bool, "Back Green"=w366:bool, "Back Blue"=w365:bool)
        n247 = Compound Arithmetic op=OR(w367, w366, w365) -> (w372:bool)
        n248 = Compound Arithmetic op=OR(w370, w369, w368) -> (w385:bool)
        n249 = Select(t=u32 16711680 ("FrontLED"), s=w367, f=u32 0 ("FrontLED")) -> (s? t:f=w377:u32)
        n250 = Select(t=u32 65280 ("FrontLED"), s=w366, f=u32 0 ("FrontLED")) -> (s? t:f=w378:u32)
        n251 = Select(t=u32 255 ("FrontLED"), s=w365, f=u32 0 ("FrontLED")) -> (s? t:f=w379:u32)
        n252 = Select(t=u32 16711680 ("FrontLED"), s=w370, f=u32 0 ("FrontLED")) -> (s? t:f=w390:u32)
        n253 = Select(t=u32 65280 ("FrontLED"), s=w369, f=u32 0 ("FrontLED")) -> (s? t:f=w391:u32)
        n254 = Select(t=u32 255 ("FrontLED"), s=w368, f=u32 0 ("FrontLED")) -> (s? t:f=w392:u32)
        n255 = call "Change Detect Boolean.vi"("In"=w372) -> ("Changed?"=w375:bool)
        n256 = call "Change Detect Boolean.vi"("In"=w385) -> ("Changed?"=w388:bool)
        n257 = And(x=w459, y=w462) -> (x .and. y?=w468:bool)
        n258 = Path To String(path="Robot Photos Folder") -> (string=w483:string)
        n259 = Compound Arithmetic op=ADD(w377, w378, w379) -> (w374:u32)
        n260 = Compound Arithmetic op=ADD(w390, w391, w392) -> (w387:u32)
        n261 = And(x=w454, y=w462) -> (x .and. y?=w467:bool)
        n262 = Select(t=u32 0, s=w375, f=w374) -> (s? t:f=→"back":u32)
        n263 = Select(t=u32 0, s=w388, f=w387) -> (s? t:f=→"front":u32)
        n264 = Concatenate Strings(w483, w464, "wings-open.png") -> (w472:string)
        n265 = Concatenate Strings(w483, w464, "hood-down.png") -> (w435:string)
        n266 = Concatenate Strings(w483, w464, "gear-flaps-open-and-traction-down.png") -> (w473:string)
        n267 = Concatenate Strings(w483, w464, "gear-flaps-open-and-h-drive-down.png") -> (w474:string)
        n268 = Concatenate Strings(w483, w464, "h-drive-down.png") -> (w432:string)
        n269 = Concatenate Strings(w483, w464, "traction-down.png") -> (w458:string)
        n270 = Concatenate Strings(w483, w464, "gear-flaps-open.png") -> (w475:string)
        n271 = Concatenate Strings(w483, w464, "original.png") -> (w476:string)
        n272 = Select(t=w475, s=w462, f=w476) -> (s? t:f=w460:string)
        n273 = Select(t=w458, s=w459, f=w460) -> (s? t:f=w456:string)
        n274 = Select(t=w432, s=w454, f=w456) -> (s? t:f=w455:string)
        n275 = Select(t=w474, s=w467, f=w455) -> (s? t:f=w470:string)
        n276 = Select(t=w473, s=w468, f=w470) -> (s? t:f=w457:string)
        n277 = Select(t=w435, s=w469, f=w457) -> (s? t:f=w461:string)
        n278 = Select(t=w472, s=w439, f=w461) -> (s? t:f=w466:string)
        n279 = String To Path(string=w466) -> (path=w465:path)
        n280 = call <vilib>:"Read PNG File.vi"("path to PNG file"=w465) -> ("image data"=w485:T65)  [unwired: 8 in, 2 out]
        n281 = call <vilib>:"Draw Flattened Pixmap.vi"("image data"=w485) -> ("new picture"=→"Robot":picture)  [unwired: 8 in]
        "Control Info" <- w536
        "Status Info" <- w535
        "Robot Metrics" <- w534
        "DS TCP" <- w533
      }
    }
  }
  n282 = while {
    tunnel: w20 -> [w573]
    tunnel: [w572] -> _
    tunnel: w18 -> [w571]
    tunnel: w19 -> [w570]
    shift-right: [w568] -> _
    shift-left: _ -> [w569]
    tunnel: w16 -> [w567]
    tunnel: w17 -> [_]
    tunnel: w15 -> [w566]
    i -> [w572]
    stop <- FALSE stop-if-true
    n283 = event shown="[0] \"Rec Mode\": Value Change" {
      selector: w571 -> [_ _ _]
      dyn-events: [w576 _ _] -> _
      timeout: _ -> [_ _ _]
      tunnel: w573 -> [w575 _ _]
      tunnel: w570 -> [_ _ _]
      tunnel: w569 -> [_ _ _]
      tunnel: [0 _ _] -> w568
      tunnel: w567 -> [_ _ w596]
      tunnel: w567 -> [w578 _ _]
      tunnel: w566 -> [w577 _ _]
      event "Rec Mode": Value Change {
        n284 = event-data() -> ("NewVal"=w579:enum32{"Stop", "Record", "Playback"})  [unwired: 1 in, 5 out]
        n285 = case shown="\"Stop\", \"Record\"" w579 {
          tunnel: w578 -> [_ w585 w591]
          tunnel: [_ _ w589] -> w576
          tunnel: cluster{i32, i32} {-250, 170} -> [_ _ w592]
          tunnel: [_ _ T66 {"Image Size"=TRUE, "Image Type"=TRUE, "Pixel Value"=TRUE, "ROI Information"=TRUE, "Zoom Factor"=FALSE} ("Image Information Shown:All Elements")] -> _
          tunnel: [_ _ TRUE ("Zoom Factor")] -> _
          tunnel: [_ _ w588] -> _
          tunnel: w577 -> [_ _ w590]
          tunnel: w575 -> [_ _ w586]
          frame Default {
          }
          frame "Stop", "Record" {
            # "Place Window too"
            n286 = invoke class="VI" method="FP.Close"(reference=w585) -> (reference out=w584:refnum<vi>)  [unwired: 2 in, 2 out]
            n287 = invoke class="VI" method="Abort VI"(reference=w584) -> ()  [unwired: 2 in, 3 out]
          }
          frame "Playback" {
            n288 = call "Open Playback Panel.vi"("Offset"=w592, "DB VI Ref"=w590, "Playback in"=w591) -> ("Playback out"=w587:refnum<vi>)  [unwired: 8 in]
            n289 = register-events(w587, w586) -> (reference out=w589:refnum<event-registration>, error out=w588:errorcluster)  [unwired: 2 in]
          }
        }
        n290 = global write "WPI_DashboardLogging Global.vi" "Logging Filename"(path "") -> ()
        n291 = global write "WPI_DashboardLogging Global.vi" "Recording"(w579) -> ()
        n292 = call <vilib>:"WPI_DashboardNT Log FieldName Cache.vi"("Operation"=enum16{"Lookup/Add", "Index", "Clear"}."Clear") -> ()  [unwired: 8 in, 3 out]
      }
      event Panel Close {
        w595 = enum32{"Stop", "Record", "Playback"}."Stop" ("Rec Mode")
        n293 = event-data() -> ()  [unwired: 1 in, 4 out]
        n294 = global write "WPI_DashboardLogging Global.vi" "Recording"(w595) -> ()
        n295 = local write "Rec Mode"(w595) -> ()
      }
      event Panel Close {
        n296 = event-data() -> ()  [unwired: 1 in, 4 out]
        n297 = invoke class="VI" method="FP.Close"(reference=w596) -> (reference out=w598:refnum<vi>)  [unwired: 2 in, 2 out]
        n298 = invoke class="VI" method="Abort VI"(reference=w598) -> (error out=w597:errorcluster)  [unwired: 2 in, 2 out]
        n299 = invoke class="VI" method="Abort VI"(error in=w597) -> ()  [unwired: 2 in, 3 out]
      }
    }
  }
  n300 = control-ref of="Dashboard Tab"() -> (w13:refnum<vi>)
  n301 = control-ref of="DumbDashMessage"() -> (w11:refnum<vi>)
  n302 = call "DumbDash Load Controls.vi"("TabControl in"=w13) -> ("Array"=w12:T67[])  [unwired: 10 in]
  n303 = global write "WPI_DashboardLogging Global.vi" "Recording"(w14) -> ()
  n304 = local write "Rec Mode"(w14) -> ()
  n305 = while {
    tunnel: w12 -> [w601]
    tunnel: w11 -> [w603]
    stop <- FALSE stop-if-true
    w602 = T69 0 items=["Main Bot", "Protobot"] ("Robot")
    n306 = First Call?() -> (First Call?: T/F=w599:bool)
    n307 = Or(x="Load", y=w599) -> (x .or. y?=w600:bool)
    n308 = case shown="True" "Save" {
      tunnel: w603 -> [_ w616]
      tunnel: w602 -> [_ w617]
      tunnel: w601 -> [_ w618]
      frame False {
      }
      frame True {
        n309 = flat-sequence {
          tunnel: w618 -> [w621]
          tunnel: w617 -> [w620]
          tunnel: w616 -> [w619]
          frame #0 {
            n310 = call "DumbDash Save Values.vi"("Message Box"=w619, "Robot"=w620, "Controls In"=w621) -> ()  [unwired: 9 in]
          }
          frame #1 {
            n311 = local write "Save"(FALSE ("Save")) -> ()
          }
        }
      }
    }
    n312 = case shown="True" w600 {
      tunnel: w603 -> [_ w611]
      tunnel: w602 -> [_ w609]
      tunnel: w601 -> [_ w610]
      frame False {
      }
      frame True {
        n313 = flat-sequence {
          tunnel: w611 -> [w614]
          tunnel: w610 -> [w613]
          tunnel: w609 -> [w612]
          frame #0 {
            n314 = call "DumbDash Load Values.vi"("Message Box"=w614, "Robot"=w612, "Controls In"=w613) -> ()  [unwired: 9 in]
          }
          frame #1 {
            n315 = local write "Load"(FALSE ("Load")) -> ()
          }
        }
      }
    }
    n316 = disable-structure shown="RUN_TIME_ENGINE==True" {
      disable-tunnel: "stop" -> [w623 w624]
      frame condition #0 (active) {
        n317 = Stop(stop? (T)=w623) -> ()
      }
      frame condition #1 {
        n318 = Quit LabVIEW(quit? (T)=w624) -> ()
      }
    }
    n319 = Wait (ms)(milliseconds to wait=u32 250) -> ()  [unwired: 1 out]
  }
